vi "final.reaction method and 1ST ziegler method).vi"() -> ()   [LabVIEW 2021]
uses:
  <vilib>/addons/Control Design/_Model Construction/Model Typedefs.llb/CD Transfer Function Model (MIMO).ctl
  <vilib>/addons/Control Design/_Model Construction/Model Typedefs.llb/CD General Elements.ctl
  <vilib>/addons/Control Design/_Model Construction/Model Typedefs.llb/CD Transfer Function Model (SISO).ctl
  <vilib>/addons/Control Design/_Model Construction/Special Model Creation.llb/Special Model Creation SubVI/CD Create PID Academic Model.vi
  <vilib>/addons/Control Design/_Dynamic Analysis/Dynamic Analysis.llb/Dynamic Analysis subVI/cd_Root Locus (Transfer Function).vi
  <vilib>/addons/Control Design/_Model Interconnection/Model Interconnection.llb/Model Interconnection SubVI/cd_Feedback (TF and TF).vi
  <vilib>/addons/Control Design/_Time Response Analysis/Time Response.llb/Time Response subVI/cd_Step Response (Transfer Function).vi
  <vilib>/addons/Control Design/_Model Construction/Model Creation.llb/Model Creation SubVI/cd_Create Transfer Function Model.vi
  <vilib>/addons/Control Design/_Model Interconnection/Model Interconnection.llb/Model Interconnection SubVI/cd_Matrix Multiply Models (TF and TF).vi
  <vilib>/addons/Control Design/_Utility/Model Viewer.llb/Model Viewer SubVI/cd_Draw Transfer Function Equation (TF).vi
  <vilib>/addons/Control Design/_Model Construction/NI_CD_Special Model Creation.lvlib
  <vilib>/addons/Control Design/_Model Interconnection/NI_CD_Model Interconnection.lvlib
  <vilib>/addons/Control Design/_Dynamic Analysis/NI_CD_Dynamic Analysis.lvlib
  <vilib>/addons/Control Design/_Time Response Analysis/NI_CD_Time Response.lvlib
  <vilib>/addons/Control Design/_Model Construction/NI_LinSys_Model Creation.lvlib
  <vilib>/addons/Control Design/_Utility/NI_CD_Model Viewer.lvlib
  <vilib>/addons/Control Design/_Model Construction/NI_LinSys_Model Typedefs.lvlib
panel:
  in  "Ti":dbl
  in  "Td":dbl
  in  "Kp":dbl
  in  "Td":dbl
  in  "Ti":dbl
  in  "Kp":dbl
  out "Root Locus G 2":cluster{dbl[], dbl[]}[](graph)=[{[], []}, {[-0.32653061224489793], [0.0]}, {[], []}, {[], []}, {array[437 elements], [0.0, 0.0, 0.0, 0.0, 0.0, 0.0, 0.0, 0.0, 0.0, 0.0, 0.0, 0.0, 0.0, 0.0, 0.0, 0.0, 0.0, 0.0, 0.0, 0.0, 0.0, 0.0, 0.0, 0.0, 0.0, 0.0, 0.0, 0.0, 0.0, 0.0, 0.0, 0.0, 0.0, 0.0, 0.0, 0.0, 0.0, 0.0, 0.0, 0.0, 0.0, 0.0, 0.0, 0.0, 0.0, 0.0, 0.0, 0.0, 0.0, 0.0, 0.0, 0.0, 0.0, 0.0, 0.0, 0.0, 0.0, 0.0, 0.0, 0.0, 0.0, 0.0, 0.0, 0.0, 0.0, 0.0, 0.0, 0.0, 0.0, 0.0, 0.0, 0.0, 0.0, 0.0, 0.0, 0.0, 0.0, 0.0, 0.0, 0.0, 0.0, 0.0, 0.0, 0.0, 0.0, 0.0, 0.0, 0.0, 0.0, 0.0, 0.0, 0.0, 0.0, 0.0, 0.0, 0.0, 0.0, 0.0, 0.0, 0.0, 0.0, 0.0, 0.0, 0.0, 0.0, 0.0, 0.0, 0.0, 0.0, 0.0, 0.0, 0.0, 0.0, 0.0, 0.0, 0.0, 0.0, 0.0, 0.0, 0.0, 0.0, 0.0, 0.0, 0.0, 0.0, 0.0, 0.0, 0.0, 0.0, 0.0, 0.0, 0.0, 0.0, 0.0, 0.0, 0.0, 0.0, 0.0, 0.0, 0.0, 0.0, 0.0, 0.0, 0.0, 0.0, 0.0, 0.0, 0.0, 0.0, 0.0, 0.0, 0.0, 0.0, 0.0, 0.0, 0.0, 0.0, 0.0, 0.0, 0.0, 0.0, 0.0, 0.0, 0.0, 0.0, 0.0, 0.0, 0.0, 0.0, 0.0, 0.0, 0.0, 0.0, 0.0, 0.0, 0.0, 0.0, 0.0, 0.0, 0.0, 0.0, 0.0, 0.0, 0.0, 0.0, 0.0, 0.0, 0.0, 0.0, 0.0, 0.0, 0.0, 0.0, 0.0, 0.0, 0.0, 0.0, 0.0, 0.0, 0.0, 0.0, 0.0, 0.0, 0.0, 0.0, 0.0, 0.0, 0.0, 0.0, 0.0, 0.0, 0.0, 0.0, 0.0, 0.0, 0.0, 0.0, 0.0, 0.0, 0.0, 0.0, 0.0, 0.0, 0.0, 0.0, 0.0, 0.0, 0.0, 0.0, 0.0, 0.0, 0.0, 0.0, 0.0, 0.0, 0.0, 0.0, 0.0, 0.0, 0.0, 0.0, 0.0, 0.0, 0.0, 0.0, 0.0, 0.0, 0.0, 0.0, 0.0, 0.0, 0.0, 0.0, 0.0, 0.0, 0.0, 0.0, 0.0, 0.0, 0.0, 0.0, 0.0, 0.0, 0.0, 0.0, 0.0, 0.0, 0.0, 0.0, 0.0, 0.0, 0.0, 0.0, 0.0, 0.0, 0.0, 0.0, 0.0, 0.0, 0.0, 0.0, 0.0, 0.0, 0.0, 0.0, 0.0, nan, nan, nan, nan, nan, nan, nan, nan, nan, nan, nan, nan, nan, nan, nan, nan, nan, nan, nan, nan, nan, nan, nan, nan, nan, nan, nan, nan, nan, nan, nan, nan, nan, nan, nan, nan, nan, nan, nan, nan, nan, nan, nan, nan, nan, nan, nan, nan, nan, nan, nan, nan, nan, nan, nan, nan, nan, nan, nan, nan, nan, nan, nan, nan, nan, nan, nan, nan, nan, nan, nan, nan, nan, nan, nan, nan, nan, nan, nan, nan, nan, nan, nan, nan, nan, nan, nan, nan, nan, nan, nan, nan, nan, nan, nan, nan, nan, nan, nan, nan, nan, nan, nan, nan, nan, nan, nan, nan, nan, nan, nan, nan, nan, nan, nan, nan, nan, nan, nan, nan, nan, nan, nan, nan, nan, nan, nan, nan, nan, nan, nan, nan, nan, nan, nan, nan, nan, nan, nan, nan, nan, nan, nan, nan, nan, nan, nan, nan, nan, nan, nan]}]
  out "Ramp Response PID  2":cluster{"time":dbl[], dbl[]}[](graph)=[{"time"=[0.0, 0.3093434343434344, 0.6186868686868688, 0.9280303030303032, 1.2373737373737377, 1.5467171717171722, 1.8560606060606064, 2.165404040404041, 2.4747474747474754, 2.7840909090909096, 3.0934343434343443, 3.4027777777777786, 3.712121212121213, 4.021464646464647, 4.330808080808082, 4.6401515151515165, 4.949494949494951, 5.258838383838385, 5.568181818181819, 5.877525252525254, 6.186868686868689, 6.496212121212123, 6.805555555555557, 7.114898989898991, 7.424242424242426, 7.733585858585861, 8.042929292929294, 8.35227272727273, 8.661616161616164, 8.970959595959599, 9.280303030303033, 9.589646464646467, 9.898989898989901, 10.208333333333336, 10.51767676767677, 10.827020202020204, 11.136363636363638, 11.445707070707073, 11.755050505050509, 12.064393939393943, 12.373737373737377], [0.0, 0.08971912221391998, 0.16317492670961967, 0.22331545284233406, 0.27255435109347836, 0.31286775133936867, 0.3458735718818212, 0.37289645219050066, 0.39502091533596234, 0.4131348937084926, 0.42796536486267295, 0.44010752767923655, 0.4500486897860373, 0.45818782492420873, 0.46485158516528746, 0.47030741060579706, 0.47477426267736766, 0.4784314118378126, 0.48142563232406227, 0.48387709271765095, 0.4858841787318348, 0.4875274417757199, 0.48887283176514507, 0.4899743439243708, 0.4908761858040183, 0.4916145514852993, 0.4922190741755815, 0.4927140154930489, 0.4931192391706285, 0.4934510082573383, 0.4937226378115482, 0.49394502928102463, 0.49412710801630716, 0.4942761814763646, 0.49439823250258136, 0.4944981594311897, 0.4945799726807021, 0.494646955704087, 0.4947017967652665, 0.4947466968285855, 0.49478345789124]}, {"time"=[0.0, 0.11874999999999998, 0.23749999999999996, 0.35624999999999996, 0.4749999999999999, 0.5937499999999999, 0.7124999999999999, 0.8312499999999998, 0.9499999999999998, 1.0687499999999999, 1.1874999999999998, 1.3062499999999997, 1.4249999999999998, 1.5437499999999997, 1.6624999999999996, 1.7812499999999998, 1.8999999999999997, 2.01875, 2.1374999999999997, 2.2562499999999996, 2.3749999999999996, 2.4937499999999995, 2.6124999999999994, 2.7312499999999997, 2.8499999999999996, 2.9687499999999996, 3.0874999999999995, 3.2062499999999994, 3.3249999999999993, 3.4437499999999996, 3.5624999999999996, 3.6812499999999995, 3.7999999999999994, 3.9187499999999993, 4.0375, 4.156249999999999, 4.2749999999999995], [0.0, 0.0, 0.0, 0.0, 0.0, 0.0, 0.0, 0.0, 0.0, 0.0, 0.0, 0.04674701942045699, 0.09781428470953771, 0.1530352107469137, 0.21224412599490042, 0.2752767774451205, 0.34197078280045506, 0.4121660332631972, 0.485705050158154, 0.562433298479174, 0.6421994603095471, 0.724855670931194, 0.8102577203047987, 0.8982652224732375, 0.9887417553140145, 1.0815549729430756, 1.1765766929524732, 1.2736829605479854, 1.3727540915400525, 1.4736746960323288, 1.5763336845467992, 1.6806242582228204, 1.786443884629593, 1.8936942606374882, 2.0022812637032796, 2.112114892837669, 2.2231092004405006]}, {"time"=[0.0, 0.01, 0.02, 0.03, 0.04, 0.05, 0.06, 0.07, 0.08, 0.09, 0.1, 0.11, 0.12, 0.13, 0.14, 0.15, 0.16, 0.17, 0.18, 0.19, 0.2, 0.21, 0.22, 0.23, 0.24, 0.25, 0.26, 0.27, 0.28, 0.29, 0.3, 0.31, 0.32, 0.33, 0.34, 0.35000000000000003, 0.36, 0.37, 0.38, 0.39, 0.4, 0.41000000000000003, 0.42, 0.43, 0.44, 0.45, 0.46, 0.47000000000000003, 0.48, 0.49, 0.5, 0.51, 0.52, 0.53, 0.54, 0.55, 0.56, 0.5700000000000001, 0.58, 0.59, 0.6, 0.61, 0.62, 0.63, 0.64, 0.65, 0.66, 0.67, 0.68, 0.6900000000000001, 0.7000000000000001, 0.71, 0.72, 0.73, 0.74, 0.75, 0.76, 0.77, 0.78, 0.79, 0.8, 0.81, 0.8200000000000001, 0.8300000000000001, 0.84, 0.85, 0.86, 0.87, 0.88, 0.89, 0.9, 0.91, 0.92, 0.93, 0.9400000000000001, 0.9500000000000001, 0.96, 0.97, 0.98, 0.99, 1.0, 1.01, 1.02, 1.03, 1.04, 1.05, 1.06, 1.07, 1.08, 1.09, 1.1, 1.11, 1.12, 1.1300000000000001, 1.1400000000000001, 1.1500000000000001, 1.16, 1.17, 1.18, 1.19, 1.2, 1.21, 1.22, 1.23, 1.24, 1.25, 1.26, 1.27, 1.28, 1.29, 1.3, 1.31, 1.32, 1.33, 1.34, 1.35, 1.36, 1.37, 1.3800000000000001, 1.3900000000000001, 1.4000000000000001, 1.41, 1.42, 1.43, 1.44, 1.45, 1.46, 1.47, 1.48, 1.49, 1.5, 1.51, 1.52, 1.53, 1.54, 1.55, 1.56, 1.57, 1.58, 1.59, 1.6, 1.61, 1.62, 1.6300000000000001, 1.6400000000000001, 1.6500000000000001, 1.6600000000000001, 1.67, 1.68, 1.69, 1.7, 1.71, 1.72, 1.73, 1.74, 1.75, 1.76, 1.77, 1.78, 1.79, 1.8, 1.81, 1.82, 1.83, 1.84, 1.85, 1.86, 1.87, 1.8800000000000001, 1.8900000000000001, 1.9000000000000001, 1.9100000000000001, 1.92, 1.93, 1.94, 1.95, 1.96, 1.97, 1.98, 1.99, 2.0, 2.0100000000000002, 2.02, 2.0300000000000002, 2.04, 2.05, 2.06, 2.07, 2.08, 2.09, 2.1, 2.11, 2.12, 2.13, 2.14, 2.15, 2.16, 2.17, 2.18, 2.19, 2.2, 2.21, 2.22, 2.23, 2.24, 2.25, 2.2600000000000002, 2.27, 2.2800000000000002, 2.29, 2.3000000000000003, 2.31, 2.32, 2.33, 2.34, 2.35, 2.36, 2.37, 2.38, 2.39, 2.4, 2.41, 2.42, 2.43, 2.44, 2.45, 2.46, 2.47, 2.48, 2.49, 2.5, 2.5100000000000002, 2.52, 2.5300000000000002, 2.54, 2.5500000000000003, 2.56, 2.57, 2.58, 2.59, 2.6, 2.61, 2.62, 2.63, 2.64, 2.65, 2.66, 2.67, 2.68, 2.69, 2.7, 2.71, 2.72, 2.73, 2.74, 2.75, 2.7600000000000002, 2.77, 2.7800000000000002, 2.79, 2.8000000000000003, 2.81, 2.82, 2.83, 2.84, 2.85, 2.86, 2.87, 2.88, 2.89, 2.9, 2.91, 2.92, 2.93, 2.94, 2.95, 2.96, 2.97, 2.98, 2.99, 3.0], [0.0, 0.01, 0.02, 0.03, 0.04, 0.05, 0.060000000000000005, 0.07, 0.08, 0.09, 0.09999999999999999, 0.10999999999999999, 0.11999999999999998, 0.12999999999999998, 0.13999999999999999, 0.15, 0.16, 0.17, 0.18000000000000002, 0.19000000000000003, 0.20000000000000004, 0.21000000000000005, 0.22000000000000006, 0.23000000000000007, 0.24000000000000007, 0.25000000000000006, 0.26000000000000006, 0.2700000000000001, 0.2800000000000001, 0.2900000000000001, 0.3000000000000001, 0.3100000000000001, 0.3200000000000001, 0.3300000000000001, 0.34000000000000014, 0.35000000000000014, 0.36000000000000015, 0.37000000000000016, 0.38000000000000017, 0.3900000000000002, 0.4000000000000002, 0.4100000000000002, 0.4200000000000002, 0.4300000000000002, 0.4400000000000002, 0.45000000000000023, 0.46000000000000024, 0.47000000000000025, 0.48000000000000026, 0.49000000000000027, 0.5000000000000002, 0.5100000000000002, 0.5200000000000002, 0.5300000000000002, 0.5400000000000003, 0.5500000000000003, 0.5600000000000003, 0.5700000000000003, 0.5800000000000003, 0.5900000000000003, 0.6000000000000003, 0.6100000000000003, 0.6200000000000003, 0.6300000000000003, 0.6400000000000003, 0.6500000000000004, 0.6600000000000004, 0.6700000000000004, 0.6800000000000004, 0.6900000000000004, 0.7000000000000004, 0.7100000000000004, 0.7200000000000004, 0.7300000000000004, 0.7400000000000004, 0.7500000000000004, 0.7600000000000005, 0.7700000000000005, 0.7800000000000005, 0.7900000000000005, 0.8000000000000005, 0.8100000000000005, 0.8200000000000005, 0.8300000000000005, 0.8400000000000005, 0.8500000000000005, 0.8600000000000005, 0.8700000000000006, 0.8800000000000006, 0.8900000000000006, 0.9000000000000006, 0.9100000000000006, 0.9200000000000006, 0.9300000000000006, 0.9400000000000006, 0.9500000000000006, 0.9600000000000006, 0.9700000000000006, 0.9800000000000006, 0.9900000000000007, 1.0000000000000007, 1.0100000000000007, 1.0200000000000007, 1.0300000000000007, 1.0400000000000007, 1.0500000000000007, 1.0600000000000007, 1.0700000000000007, 1.0800000000000007, 1.0900000000000007, 1.1000000000000008, 1.1100000000000008, 1.1200000000000008, 1.1300000000000008, 1.1400000000000008, 1.1500000000000008, 1.1600000000000008, 1.1700000000000008, 1.1800000000000008, 1.1900000000000008, 1.2000000000000008, 1.2100000000000009, 1.2200000000000009, 1.2300000000000009, 1.2400000000000009, 1.2500000000000009, 1.260000000000001, 1.270000000000001, 1.280000000000001, 1.290000000000001, 1.300000000000001, 1.310000000000001, 1.320000000000001, 1.330000000000001, 1.340000000000001, 1.350000000000001, 1.360000000000001, 1.370000000000001, 1.380000000000001, 1.390000000000001, 1.400000000000001, 1.410000000000001, 1.420000000000001, 1.430000000000001, 1.440000000000001, 1.450000000000001, 1.460000000000001, 1.470000000000001, 1.480000000000001, 1.490000000000001, 1.500000000000001, 1.5100000000000011, 1.5200000000000011, 1.5300000000000011, 1.5400000000000011, 1.5500000000000012, 1.5600000000000012, 1.5700000000000012, 1.5800000000000012, 1.5900000000000012, 1.6000000000000012, 1.6100000000000012, 1.6200000000000012, 1.6300000000000012, 1.6400000000000012, 1.6500000000000012, 1.6600000000000013, 1.6700000000000013, 1.6800000000000013, 1.6900000000000013, 1.7000000000000013, 1.7100000000000013, 1.7200000000000013, 1.7300000000000013, 1.7400000000000013, 1.7500000000000013, 1.7600000000000013, 1.7700000000000014, 1.7800000000000014, 1.7900000000000014, 1.8000000000000014, 1.8100000000000014, 1.8200000000000014, 1.8300000000000014, 1.8400000000000014, 1.8500000000000014, 1.8600000000000014, 1.8700000000000014, 1.8800000000000014, 1.8900000000000015, 1.9000000000000015, 1.9100000000000015, 1.9200000000000015, 1.9300000000000015, 1.9400000000000015, 1.9500000000000015, 1.9600000000000015, 1.9700000000000015, 1.9800000000000015, 1.9900000000000015, 2.0000000000000013, 2.010000000000001, 2.020000000000001, 2.0300000000000007, 2.0400000000000005, 2.0500000000000003, 2.06, 2.07, 2.0799999999999996, 2.0899999999999994, 2.099999999999999, 2.109999999999999, 2.1199999999999988, 2.1299999999999986, 2.1399999999999983, 2.149999999999998, 2.159999999999998, 2.1699999999999977, 2.1799999999999975, 2.1899999999999973, 2.199999999999997, 2.209999999999997, 2.2199999999999966, 2.2299999999999964, 2.239999999999996, 2.249999999999996, 2.259999999999996, 2.2699999999999956, 2.2799999999999954, 2.289999999999995, 2.299999999999995, 2.3099999999999947, 2.3199999999999945, 2.3299999999999943, 2.339999999999994, 2.349999999999994, 2.3599999999999937, 2.3699999999999934, 2.3799999999999932, 2.389999999999993, 2.399999999999993, 2.4099999999999926, 2.4199999999999924, 2.429999999999992, 2.439999999999992, 2.4499999999999917, 2.4599999999999915, 2.4699999999999913, 2.479999999999991, 2.489999999999991, 2.4999999999999907, 2.5099999999999905, 2.5199999999999902, 2.52999999999999, 2.53999999999999, 2.5499999999999896, 2.5599999999999894, 2.569999999999989, 2.579999999999989, 2.5899999999999888, 2.5999999999999885, 2.6099999999999883, 2.619999999999988, 2.629999999999988, 2.6399999999999877, 2.6499999999999875, 2.6599999999999873, 2.669999999999987, 2.679999999999987, 2.6899999999999866, 2.6999999999999864, 2.709999999999986, 2.719999999999986, 2.7299999999999858, 2.7399999999999856, 2.7499999999999853, 2.759999999999985, 2.769999999999985, 2.7799999999999847, 2.7899999999999845, 2.7999999999999843, 2.809999999999984, 2.819999999999984, 2.8299999999999836, 2.8399999999999834, 2.849999999999983, 2.859999999999983, 2.869999999999983, 2.8799999999999826, 2.8899999999999824, 2.899999999999982, 2.909999999999982, 2.9199999999999817, 2.9299999999999815, 2.9399999999999813, 2.949999999999981, 2.959999999999981, 2.9699999999999807, 2.9799999999999804, 2.9899999999999802, 2.99999999999998]}]
  out "Step Response PID 2":cluster{"time":dbl[], dbl[]}[](graph)=[{"time"=[0.0, 0.3093434343434344, 0.6186868686868688, 0.9280303030303032, 1.2373737373737377, 1.5467171717171722, 1.8560606060606064, 2.165404040404041, 2.4747474747474754, 2.7840909090909096, 3.0934343434343443, 3.4027777777777786, 3.712121212121213, 4.021464646464647, 4.330808080808082, 4.6401515151515165, 4.949494949494951, 5.258838383838385, 5.568181818181819, 5.877525252525254, 6.186868686868689, 6.496212121212123, 6.805555555555557, 7.114898989898991, 7.424242424242426, 7.733585858585861, 8.042929292929294, 8.35227272727273, 8.661616161616164, 8.970959595959599, 9.280303030303033, 9.589646464646467, 9.898989898989901, 10.208333333333336, 10.51767676767677, 10.827020202020204, 11.136363636363638, 11.445707070707073, 11.755050505050509, 12.064393939393943, 12.373737373737377], [0.0, 0.08971912221391998, 0.16317492670961967, 0.22331545284233406, 0.27255435109347836, 0.31286775133936867, 0.3458735718818212, 0.37289645219050066, 0.39502091533596234, 0.4131348937084926, 0.42796536486267295, 0.44010752767923655, 0.4500486897860373, 0.45818782492420873, 0.46485158516528746, 0.47030741060579706, 0.47477426267736766, 0.4784314118378126, 0.48142563232406227, 0.48387709271765095, 0.4858841787318348, 0.4875274417757199, 0.48887283176514507, 0.4899743439243708, 0.4908761858040183, 0.4916145514852993, 0.4922190741755815, 0.4927140154930489, 0.4931192391706285, 0.4934510082573383, 0.4937226378115482, 0.49394502928102463, 0.49412710801630716, 0.4942761814763646, 0.49439823250258136, 0.4944981594311897, 0.4945799726807021, 0.494646955704087, 0.4947017967652665, 0.4947466968285855, 0.49478345789124]}, {"time"=[0.0, 0.11874999999999998, 0.23749999999999996, 0.35624999999999996, 0.4749999999999999, 0.5937499999999999, 0.7124999999999999, 0.8312499999999998, 0.9499999999999998, 1.0687499999999999, 1.1874999999999998, 1.3062499999999997, 1.4249999999999998, 1.5437499999999997, 1.6624999999999996, 1.7812499999999998, 1.8999999999999997, 2.01875, 2.1374999999999997, 2.2562499999999996, 2.3749999999999996, 2.4937499999999995, 2.6124999999999994, 2.7312499999999997, 2.8499999999999996, 2.9687499999999996, 3.0874999999999995, 3.2062499999999994, 3.3249999999999993, 3.4437499999999996, 3.5624999999999996, 3.6812499999999995, 3.7999999999999994, 3.9187499999999993, 4.0375, 4.156249999999999, 4.2749999999999995, 4.393749999999999, 4.512499999999999, 4.63125, 4.749999999999999, 4.8687499999999995, 4.987499999999999, 5.106249999999999, 5.224999999999999, 5.343749999999999, 5.4624999999999995, 5.581249999999999, 5.699999999999999, 5.818749999999999, 5.937499999999999, 6.056249999999999, 6.174999999999999, 6.293749999999999, 6.412499999999999, 6.531249999999999, 6.649999999999999, 6.768749999999999, 6.887499999999999, 7.006249999999999, 7.124999999999999, 7.243749999999999, 7.362499999999999, 7.481249999999998, 7.599999999999999, 7.718749999999999, 7.837499999999999, 7.956249999999999, 8.075, 8.193749999999998, 8.312499999999998, 8.431249999999999, 8.549999999999999, 8.66875, 8.787499999999998, 8.906249999999998, 9.024999999999999, 9.143749999999999, 9.2625, 9.381249999999998, 9.499999999999998, 9.618749999999999, 9.737499999999999, 9.856249999999998, 9.974999999999998, 10.093749999999998, 10.212499999999999, 10.331249999999999, 10.449999999999998, 10.568749999999998, 10.687499999999998, 10.806249999999999, 10.924999999999999, 11.043749999999998, 11.162499999999998, 11.281249999999998, 11.399999999999999, 11.518749999999999, 11.637499999999998, 11.756249999999998, 11.874999999999998, 11.993749999999999, 12.112499999999997, 12.231249999999998, 12.349999999999998, 12.468749999999998, 12.587499999999999, 12.706249999999997, 12.824999999999998, 12.943749999999998, 13.062499999999998, 13.181249999999999, 13.299999999999997, 13.418749999999998, 13.537499999999998, 13.656249999999998, 13.774999999999999, 13.893749999999997, 14.012499999999998, 14.131249999999998, 14.249999999999998, 14.368749999999997, 14.487499999999997, 14.606249999999998, 14.724999999999998, 14.843749999999998, 14.962499999999997, 15.081249999999997, 15.199999999999998, 15.318749999999998, 15.437499999999998, 15.556249999999997, 15.674999999999997, 15.793749999999998, 15.912499999999998, 16.031249999999996, 16.15, 16.268749999999997, 16.387499999999996, 16.506249999999998, 16.624999999999996, 16.74375, 16.862499999999997, 16.981249999999996, 17.099999999999998, 17.218749999999996, 17.3375, 17.456249999999997, 17.574999999999996, 17.693749999999998, 17.812499999999996, 17.93125, 18.049999999999997, 18.168749999999996, 18.287499999999998, 18.406249999999996, 18.525, 18.643749999999997, 18.762499999999996, 18.881249999999998, 18.999999999999996, 19.11875, 19.237499999999997, 19.356249999999996, 19.474999999999998, 19.593749999999996, 19.712499999999995, 19.831249999999997, 19.949999999999996, 20.068749999999998, 20.187499999999996, 20.306249999999995, 20.424999999999997], [0.0, 0.0, 0.0, 0.0, 0.0, 0.0, 0.0, 0.0, 0.0, 0.0, 0.37499999999999994, 0.41208383650020264, 0.4477625386272583, 0.4820415181676434, 0.5149306710217187, 0.546443918273478, 0.5765987762501894, 0.60541595436764, 0.6329189795713029, 0.659133846201218, 0.6840886901283811, 0.7078134860326692, 0.7303397667164837, 0.7517003633741237, 0.7719291657641358, 0.7910609012603143, 0.8091309317864142, 0.826175067669815, 0.8422293974801205, 0.8573301329498857, 0.871513468106107, 0.8848154517727276, 0.8972718726360158, 0.9089181560961823, 0.9197892721599139, 0.9299196536595047, 0.9393431241148937, 0.9480928345850927, 0.9562012088851455, 0.9636998965738381, 0.9706197331458364, 0.9769907068897197, 0.9828419319004598, 0.9882016267612508, 0.9930970984351859, 0.9975547309321007, 1.0015999783399123, 1.005257361833018, 1.008550470292714, 1.0115019641961918, 1.014133582451457, 1.0164661518754707, 1.018519599031985, 1.0203129641639086, 1.0218644169726037, 1.0231912740133304, 1.0243100174920705, 1.0252363152642676, 1.025985041850562, 1.0265703002984465, 1.027005444731907, 1.027303103443579, 1.0274752023957554, 1.0275329890077547, 1.0274870561176976, 1.0273473660167067, 1.027123274462909, 1.0268235545914517, 1.0264564206450182, 1.0260295514571196, 1.0255501136277019, 1.0250247843374294, 1.0244597737533598, 1.0238608469846466, 1.0232333455524238, 1.0225822083431462, 1.0219119920194026, 1.021226890866614, 1.020530756058076, 1.0198271143245452, 1.0191191860179887, 1.0184099025622688, 1.0177019232863962, 1.016997651638608, 1.0162992507818982, 1.0156086585737762, 1.014927601934967, 1.014257610613496, 1.0136000303521622, 1.0129560354687606, 1.0123266408596414, 1.0117127134382407, 1.0111149830211406, 1.0105340526749993, 1.0099704085383578, 1.0094244291328764, 1.0088963941790066, 1.008386492931452, 1.0078948320500378, 1.007421443021783, 1.006966289150093, 1.0065292721270185, 1.006110238204514, 1.0057089839805538, 1.0053252618158426, 1.004958784896684, 1.0046092319593687, 1.0042762516911932, 1.0039594668229592, 1.0036584779274862, 1.0033728669383584, 1.0031022004027752, 1.002846032482018, 1.0026039077126674, 1.0023753635413133, 1.00215993264512, 1.0019571450501852, 1.00176653005924, 1.0015876179998215, 1.0014199418036387, 1.0012630384274408, 1.0011164501252932, 1.0009797255817554, 1.000852420915059, 1.0007341005589863, 1.0006243380317605, 1.00052271659988, 1.0004288298444477, 1.0003422821371901, 1.0002626890329978, 1.0001896775854693, 1.0001228865916116, 1.0000619667715123, 1.0000065808884857, 0.9999564038148911, 0.9999111225485162, 0.9998704361841395, 0.9998340558446084, 0.9998017045755001, 0.9997731172071864, 0.9997480401878693, 0.9997262313909276, 0.9997074598996916, 0.9996915057725395, 0.9996781597910218, 0.9996672231935075, 0.9996585073966762, 0.9996518337069942, 0.999647033024156, 0.9996439455383013, 0.9996424204226821, 0.9996423155233032, 0.9996434970469326, 0.9996458392487444, 0.9996492241207497, 0.9996535410820484, 0.9996586866718364, 0.9996645642460062, 0.9996710836780791, 0.9996781610651322, 0.9996857184392944, 0.9996936834853181, 0.9997019892646546, 0.9997105739464132, 0.9997193805455022, 0.9997283566682198, 0.9997374542654873, 0.9997466293938946, 0.9997558419846626, 0.999765055620607, 0.9997742373211389, 0.9997833573353125, 0.9997923889428968]}, {"time"=[0.0, 0.01, 0.02, 0.03, 0.04, 0.05, 0.06, 0.07, 0.08, 0.09, 0.1, 0.11, 0.12, 0.13, 0.14, 0.15, 0.16, 0.17, 0.18, 0.19, 0.2, 0.21, 0.22, 0.23, 0.24, 0.25, 0.26, 0.27, 0.28, 0.29, 0.3, 0.31, 0.32, 0.33, 0.34, 0.35000000000000003, 0.36, 0.37, 0.38, 0.39, 0.4, 0.41000000000000003, 0.42, 0.43, 0.44, 0.45, 0.46, 0.47000000000000003, 0.48, 0.49, 0.5, 0.51, 0.52, 0.53, 0.54, 0.55, 0.56, 0.5700000000000001, 0.58, 0.59, 0.6, 0.61, 0.62, 0.63, 0.64, 0.65, 0.66, 0.67, 0.68, 0.6900000000000001, 0.7000000000000001, 0.71, 0.72, 0.73, 0.74, 0.75, 0.76, 0.77, 0.78, 0.79, 0.8, 0.81, 0.8200000000000001, 0.8300000000000001, 0.84, 0.85, 0.86, 0.87, 0.88, 0.89, 0.9, 0.91, 0.92, 0.93, 0.9400000000000001, 0.9500000000000001, 0.96, 0.97, 0.98, 0.99, 1.0, 1.01, 1.02, 1.03, 1.04, 1.05, 1.06, 1.07, 1.08, 1.09, 1.1, 1.11, 1.12, 1.1300000000000001, 1.1400000000000001, 1.1500000000000001, 1.16, 1.17, 1.18, 1.19, 1.2, 1.21, 1.22, 1.23, 1.24, 1.25, 1.26, 1.27, 1.28, 1.29, 1.3, 1.31, 1.32, 1.33, 1.34, 1.35, 1.36, 1.37, 1.3800000000000001, 1.3900000000000001, 1.4000000000000001, 1.41, 1.42, 1.43, 1.44, 1.45, 1.46, 1.47, 1.48, 1.49, 1.5, 1.51, 1.52, 1.53, 1.54, 1.55, 1.56, 1.57, 1.58, 1.59, 1.6, 1.61, 1.62, 1.6300000000000001, 1.6400000000000001, 1.6500000000000001, 1.6600000000000001, 1.67, 1.68, 1.69, 1.7, 1.71, 1.72, 1.73, 1.74, 1.75, 1.76, 1.77, 1.78, 1.79, 1.8, 1.81, 1.82, 1.83, 1.84, 1.85, 1.86, 1.87, 1.8800000000000001, 1.8900000000000001, 1.9000000000000001, 1.9100000000000001, 1.92, 1.93, 1.94, 1.95, 1.96, 1.97, 1.98, 1.99, 2.0, 2.0100000000000002, 2.02, 2.0300000000000002, 2.04, 2.05, 2.06, 2.07, 2.08, 2.09, 2.1, 2.11, 2.12, 2.13, 2.14, 2.15, 2.16, 2.17, 2.18, 2.19, 2.2, 2.21, 2.22, 2.23, 2.24, 2.25, 2.2600000000000002, 2.27, 2.2800000000000002, 2.29, 2.3000000000000003, 2.31, 2.32, 2.33, 2.34, 2.35, 2.36, 2.37, 2.38, 2.39, 2.4, 2.41, 2.42, 2.43, 2.44, 2.45, 2.46, 2.47, 2.48, 2.49, 2.5, 2.5100000000000002, 2.52, 2.5300000000000002, 2.54, 2.5500000000000003, 2.56, 2.57, 2.58, 2.59, 2.6, 2.61, 2.62, 2.63, 2.64, 2.65, 2.66, 2.67, 2.68, 2.69, 2.7, 2.71, 2.72, 2.73, 2.74, 2.75, 2.7600000000000002, 2.77, 2.7800000000000002, 2.79, 2.8000000000000003, 2.81, 2.82, 2.83, 2.84, 2.85, 2.86, 2.87, 2.88, 2.89, 2.9, 2.91, 2.92, 2.93, 2.94, 2.95, 2.96, 2.97, 2.98, 2.99, 3.0], [1.0, 1.0, 1.0, 1.0, 1.0, 1.0, 1.0, 1.0, 1.0, 1.0, 1.0, 1.0, 1.0, 1.0, 1.0, 1.0, 1.0, 1.0, 1.0, 1.0, 1.0, 1.0, 1.0, 1.0, 1.0, 1.0, 1.0, 1.0, 1.0, 1.0, 1.0, 1.0, 1.0, 1.0, 1.0, 1.0, 1.0, 1.0, 1.0, 1.0, 1.0, 1.0, 1.0, 1.0, 1.0, 1.0, 1.0, 1.0, 1.0, 1.0, 1.0, 1.0, 1.0, 1.0, 1.0, 1.0, 1.0, 1.0, 1.0, 1.0, 1.0, 1.0, 1.0, 1.0, 1.0, 1.0, 1.0, 1.0, 1.0, 1.0, 1.0, 1.0, 1.0, 1.0, 1.0, 1.0, 1.0, 1.0, 1.0, 1.0, 1.0, 1.0, 1.0, 1.0, 1.0, 1.0, 1.0, 1.0, 1.0, 1.0, 1.0, 1.0, 1.0, 1.0, 1.0, 1.0, 1.0, 1.0, 1.0, 1.0, 1.0, 1.0, 1.0, 1.0, 1.0, 1.0, 1.0, 1.0, 1.0, 1.0, 1.0, 1.0, 1.0, 1.0, 1.0, 1.0, 1.0, 1.0, 1.0, 1.0, 1.0, 1.0, 1.0, 1.0, 1.0, 1.0, 1.0, 1.0, 1.0, 1.0, 1.0, 1.0, 1.0, 1.0, 1.0, 1.0, 1.0, 1.0, 1.0, 1.0, 1.0, 1.0, 1.0, 1.0, 1.0, 1.0, 1.0, 1.0, 1.0, 1.0, 1.0, 1.0, 1.0, 1.0, 1.0, 1.0, 1.0, 1.0, 1.0, 1.0, 1.0, 1.0, 1.0, 1.0, 1.0, 1.0, 1.0, 1.0, 1.0, 1.0, 1.0, 1.0, 1.0, 1.0, 1.0, 1.0, 1.0, 1.0, 1.0, 1.0, 1.0, 1.0, 1.0, 1.0, 1.0, 1.0, 1.0, 1.0, 1.0, 1.0, 1.0, 1.0, 1.0, 1.0, 1.0, 1.0, 1.0, 1.0, 1.0, 1.0, 1.0, 1.0, 1.0, 1.0, 1.0, 1.0, 1.0, 1.0, 1.0, 1.0, 1.0, 1.0, 1.0, 1.0, 1.0, 1.0, 1.0, 1.0, 1.0, 1.0, 1.0, 1.0, 1.0, 1.0, 1.0, 1.0, 1.0, 1.0, 1.0, 1.0, 1.0, 1.0, 1.0, 1.0, 1.0, 1.0, 1.0, 1.0, 1.0, 1.0, 1.0, 1.0, 1.0, 1.0, 1.0, 1.0, 1.0, 1.0, 1.0, 1.0, 1.0, 1.0, 1.0, 1.0, 1.0, 1.0, 1.0, 1.0, 1.0, 1.0, 1.0, 1.0, 1.0, 1.0, 1.0, 1.0, 1.0, 1.0, 1.0, 1.0, 1.0, 1.0, 1.0, 1.0, 1.0, 1.0, 1.0, 1.0, 1.0, 1.0, 1.0, 1.0, 1.0, 1.0, 1.0, 1.0, 1.0, 1.0, 1.0, 1.0, 1.0, 1.0, 1.0, 1.0, 1.0, 1.0, 1.0, 1.0, 1.0, 1.0, 1.0]}]
  out "Root Locus PID 2":cluster{dbl[], dbl[]}[](graph)=[{[], []}, {[-0.32653061224489793, 0.0], [0.0, 0.0]}, {[-0.8421052631578949, -0.8421052631578949], [1.1468530207045996e-08, -1.1468530207045996e-08]}, {[-0.20253164556962014], [0.0]}, {array[413 elements], array[413 elements]}, {array[413 elements], array[413 elements]}]
  out "Equation":picture
  out "open loop step response":cluster{"time":dbl[], dbl[]}[](graph)=[{"time"=array[218 elements], array[218 elements]}, {"time"=[0.0, 0.01, 0.02, 0.03, 0.04, 0.05, 0.06, 0.07, 0.08, 0.09, 0.1, 0.11, 0.12, 0.13, 0.14, 0.15, 0.16, 0.17, 0.18, 0.19, 0.2, 0.21, 0.22, 0.23, 0.24, 0.25, 0.26, 0.27, 0.28, 0.29, 0.3, 0.31, 0.32, 0.33, 0.34, 0.35000000000000003, 0.36, 0.37, 0.38, 0.39, 0.4, 0.41000000000000003, 0.42, 0.43, 0.44, 0.45, 0.46, 0.47000000000000003, 0.48, 0.49, 0.5, 0.51, 0.52, 0.53, 0.54, 0.55, 0.56, 0.5700000000000001, 0.58, 0.59, 0.6, 0.61, 0.62, 0.63, 0.64, 0.65, 0.66, 0.67, 0.68, 0.6900000000000001, 0.7000000000000001, 0.71, 0.72, 0.73, 0.74, 0.75, 0.76, 0.77, 0.78, 0.79, 0.8, 0.81, 0.8200000000000001, 0.8300000000000001, 0.84, 0.85, 0.86, 0.87, 0.88, 0.89, 0.9, 0.91, 0.92, 0.93, 0.9400000000000001, 0.9500000000000001, 0.96, 0.97, 0.98, 0.99, 1.0, 1.01, 1.02, 1.03, 1.04, 1.05, 1.06, 1.07, 1.08, 1.09, 1.1, 1.11, 1.12, 1.1300000000000001, 1.1400000000000001, 1.1500000000000001, 1.16, 1.17, 1.18, 1.19, 1.2, 1.21, 1.22, 1.23, 1.24, 1.25, 1.26, 1.27, 1.28, 1.29, 1.3, 1.31, 1.32, 1.33, 1.34, 1.35, 1.36, 1.37, 1.3800000000000001, 1.3900000000000001, 1.4000000000000001, 1.41, 1.42, 1.43, 1.44, 1.45, 1.46, 1.47, 1.48, 1.49, 1.5, 1.51, 1.52, 1.53, 1.54, 1.55, 1.56, 1.57, 1.58, 1.59, 1.6, 1.61, 1.62, 1.6300000000000001, 1.6400000000000001, 1.6500000000000001, 1.6600000000000001, 1.67, 1.68, 1.69, 1.7, 1.71, 1.72, 1.73, 1.74, 1.75, 1.76, 1.77, 1.78, 1.79, 1.8, 1.81, 1.82, 1.83, 1.84, 1.85, 1.86, 1.87, 1.8800000000000001, 1.8900000000000001, 1.9000000000000001, 1.9100000000000001, 1.92, 1.93, 1.94, 1.95, 1.96, 1.97, 1.98, 1.99, 2.0, 2.0100000000000002, 2.02, 2.0300000000000002, 2.04, 2.05, 2.06, 2.07, 2.08, 2.09, 2.1, 2.11, 2.12, 2.13, 2.14, 2.15, 2.16, 2.17, 2.18, 2.19, 2.2, 2.21, 2.22, 2.23, 2.24, 2.25, 2.2600000000000002, 2.27, 2.2800000000000002, 2.29, 2.3000000000000003, 2.31, 2.32, 2.33, 2.34, 2.35, 2.36, 2.37, 2.38, 2.39, 2.4, 2.41, 2.42, 2.43, 2.44, 2.45, 2.46, 2.47, 2.48, 2.49, 2.5, 2.5100000000000002, 2.52, 2.5300000000000002, 2.54, 2.5500000000000003, 2.56, 2.57, 2.58, 2.59, 2.6, 2.61, 2.62, 2.63, 2.64, 2.65, 2.66, 2.67, 2.68, 2.69, 2.7, 2.71, 2.72, 2.73, 2.74, 2.75, 2.7600000000000002, 2.77, 2.7800000000000002, 2.79, 2.8000000000000003, 2.81, 2.82, 2.83, 2.84, 2.85, 2.86, 2.87, 2.88, 2.89, 2.9, 2.91, 2.92, 2.93, 2.94, 2.95, 2.96, 2.97, 2.98, 2.99, 3.0], [1.0, 1.0, 1.0, 1.0, 1.0, 1.0, 1.0, 1.0, 1.0, 1.0, 1.0, 1.0, 1.0, 1.0, 1.0, 1.0, 1.0, 1.0, 1.0, 1.0, 1.0, 1.0, 1.0, 1.0, 1.0, 1.0, 1.0, 1.0, 1.0, 1.0, 1.0, 1.0, 1.0, 1.0, 1.0, 1.0, 1.0, 1.0, 1.0, 1.0, 1.0, 1.0, 1.0, 1.0, 1.0, 1.0, 1.0, 1.0, 1.0, 1.0, 1.0, 1.0, 1.0, 1.0, 1.0, 1.0, 1.0, 1.0, 1.0, 1.0, 1.0, 1.0, 1.0, 1.0, 1.0, 1.0, 1.0, 1.0, 1.0, 1.0, 1.0, 1.0, 1.0, 1.0, 1.0, 1.0, 1.0, 1.0, 1.0, 1.0, 1.0, 1.0, 1.0, 1.0, 1.0, 1.0, 1.0, 1.0, 1.0, 1.0, 1.0, 1.0, 1.0, 1.0, 1.0, 1.0, 1.0, 1.0, 1.0, 1.0, 1.0, 1.0, 1.0, 1.0, 1.0, 1.0, 1.0, 1.0, 1.0, 1.0, 1.0, 1.0, 1.0, 1.0, 1.0, 1.0, 1.0, 1.0, 1.0, 1.0, 1.0, 1.0, 1.0, 1.0, 1.0, 1.0, 1.0, 1.0, 1.0, 1.0, 1.0, 1.0, 1.0, 1.0, 1.0, 1.0, 1.0, 1.0, 1.0, 1.0, 1.0, 1.0, 1.0, 1.0, 1.0, 1.0, 1.0, 1.0, 1.0, 1.0, 1.0, 1.0, 1.0, 1.0, 1.0, 1.0, 1.0, 1.0, 1.0, 1.0, 1.0, 1.0, 1.0, 1.0, 1.0, 1.0, 1.0, 1.0, 1.0, 1.0, 1.0, 1.0, 1.0, 1.0, 1.0, 1.0, 1.0, 1.0, 1.0, 1.0, 1.0, 1.0, 1.0, 1.0, 1.0, 1.0, 1.0, 1.0, 1.0, 1.0, 1.0, 1.0, 1.0, 1.0, 1.0, 1.0, 1.0, 1.0, 1.0, 1.0, 1.0, 1.0, 1.0, 1.0, 1.0, 1.0, 1.0, 1.0, 1.0, 1.0, 1.0, 1.0, 1.0, 1.0, 1.0, 1.0, 1.0, 1.0, 1.0, 1.0, 1.0, 1.0, 1.0, 1.0, 1.0, 1.0, 1.0, 1.0, 1.0, 1.0, 1.0, 1.0, 1.0, 1.0, 1.0, 1.0, 1.0, 1.0, 1.0, 1.0, 1.0, 1.0, 1.0, 1.0, 1.0, 1.0, 1.0, 1.0, 1.0, 1.0, 1.0, 1.0, 1.0, 1.0, 1.0, 1.0, 1.0, 1.0, 1.0, 1.0, 1.0, 1.0, 1.0, 1.0, 1.0, 1.0, 1.0, 1.0, 1.0, 1.0, 1.0, 1.0, 1.0, 1.0, 1.0, 1.0, 1.0, 1.0, 1.0, 1.0, 1.0, 1.0, 1.0, 1.0, 1.0, 1.0, 1.0, 1.0, 1.0, 1.0, 1.0, 1.0, 1.0, 1.0, 1.0, 1.0, 1.0, 1.0, 1.0, 1.0, 1.0]}]
  in  "Td":dbl
  in  "Kp":dbl
  in  "Pcr":dbl
  in  "Kcr":dbl
  in  "choose 2":string(combo)
  out "Root Locus G":cluster{dbl[], dbl[]}[](graph)
  out "Ramp Response PID":cluster{"time":dbl[], dbl[]}[](graph)=[{"time"=[0.0, 0.01, 0.02, 0.03, 0.04, 0.05, 0.06, 0.07, 0.08, 0.09, 0.1, 0.11, 0.12, 0.13, 0.14, 0.15, 0.16, 0.17, 0.18, 0.19, 0.2, 0.21, 0.22, 0.23, 0.24, 0.25, 0.26, 0.27, 0.28, 0.29, 0.3, 0.31, 0.32, 0.33, 0.34, 0.35000000000000003, 0.36, 0.37, 0.38, 0.39, 0.4, 0.41000000000000003, 0.42, 0.43, 0.44, 0.45, 0.46, 0.47000000000000003, 0.48, 0.49, 0.5, 0.51, 0.52, 0.53, 0.54, 0.55, 0.56, 0.5700000000000001, 0.58, 0.59, 0.6, 0.61, 0.62, 0.63, 0.64, 0.65, 0.66, 0.67, 0.68, 0.6900000000000001, 0.7000000000000001, 0.71, 0.72, 0.73, 0.74, 0.75, 0.76, 0.77, 0.78, 0.79, 0.8, 0.81, 0.8200000000000001, 0.8300000000000001, 0.84, 0.85, 0.86, 0.87, 0.88, 0.89, 0.9, 0.91, 0.92, 0.93, 0.9400000000000001, 0.9500000000000001, 0.96, 0.97, 0.98, 0.99, 1.0, 1.01, 1.02, 1.03, 1.04, 1.05, 1.06, 1.07, 1.08, 1.09, 1.1, 1.11, 1.12, 1.1300000000000001, 1.1400000000000001, 1.1500000000000001, 1.16, 1.17, 1.18, 1.19, 1.2, 1.21, 1.22, 1.23, 1.24, 1.25, 1.26, 1.27, 1.28, 1.29, 1.3, 1.31, 1.32, 1.33, 1.34, 1.35, 1.36, 1.37, 1.3800000000000001, 1.3900000000000001, 1.4000000000000001, 1.41, 1.42, 1.43, 1.44, 1.45, 1.46, 1.47, 1.48, 1.49, 1.5, 1.51, 1.52, 1.53, 1.54, 1.55, 1.56, 1.57, 1.58, 1.59, 1.6, 1.61, 1.62, 1.6300000000000001, 1.6400000000000001, 1.6500000000000001, 1.6600000000000001, 1.67, 1.68, 1.69, 1.7, 1.71, 1.72, 1.73, 1.74, 1.75, 1.76, 1.77, 1.78, 1.79, 1.8, 1.81, 1.82, 1.83, 1.84, 1.85, 1.86, 1.87, 1.8800000000000001, 1.8900000000000001, 1.9000000000000001, 1.9100000000000001, 1.92, 1.93, 1.94, 1.95, 1.96, 1.97, 1.98, 1.99, 2.0, 2.0100000000000002, 2.02, 2.0300000000000002, 2.04, 2.05, 2.06, 2.07, 2.08, 2.09, 2.1, 2.11, 2.12, 2.13, 2.14, 2.15, 2.16, 2.17, 2.18, 2.19, 2.2, 2.21, 2.22, 2.23, 2.24, 2.25, 2.2600000000000002, 2.27, 2.2800000000000002, 2.29, 2.3000000000000003, 2.31, 2.32, 2.33, 2.34, 2.35, 2.36, 2.37, 2.38, 2.39, 2.4, 2.41, 2.42, 2.43, 2.44, 2.45, 2.46, 2.47, 2.48, 2.49, 2.5, 2.5100000000000002, 2.52, 2.5300000000000002, 2.54, 2.5500000000000003, 2.56, 2.57, 2.58, 2.59, 2.6, 2.61, 2.62, 2.63, 2.64, 2.65, 2.66, 2.67, 2.68, 2.69, 2.7, 2.71, 2.72, 2.73, 2.74, 2.75, 2.7600000000000002, 2.77, 2.7800000000000002, 2.79, 2.8000000000000003, 2.81, 2.82, 2.83, 2.84, 2.85, 2.86, 2.87, 2.88, 2.89, 2.9, 2.91, 2.92, 2.93, 2.94, 2.95, 2.96, 2.97, 2.98, 2.99, 3.0], [0.0, 0.0, 0.0, 0.0, 0.0, 0.0, 0.0, 0.0, 0.0, 0.0, 0.0, 0.0, 0.0, 0.0, 0.0, 0.0, 0.0, 0.0, 0.0, 0.0, 0.0, 0.0, 0.0, 0.0, 0.0, 0.0, 0.0, 0.0, 0.0, 0.0, 0.0, 0.0, 0.0, 0.0, 0.0, 0.0, 0.0, 0.0, 0.0, 0.0, 0.0, 0.0, 0.0, 0.0, 0.0, 0.0, 0.0, 0.0, 0.0, 0.0, 0.0, 0.0, 0.0, 0.0, 0.0, 0.0, 0.0, 0.0, 0.0, 0.0, 0.0, 0.0, 0.0, 0.0, 0.0, 0.0, 0.0, 0.0, 0.0, 0.0, 0.0, 0.0, 0.0, 0.0, 0.0, 0.0, 0.0, 0.0, 0.0, 0.0, 0.0, 0.0, 0.0, 0.0, 0.0, 0.0, 0.0, 0.0, 0.0, 0.0, 0.0, 0.0, 0.0, 0.0, 0.0, 0.0, 0.0, 0.0, 0.0, 0.0, 0.0, 0.0, 0.0, 0.0, 0.0, 0.0, 0.0, 0.0, 0.0, 0.0, 0.0, 0.0, 0.0, 0.0, 0.0, 0.0, 0.0, 0.0, 0.0, 0.0, 0.0, 0.0, 0.0, 0.0, 0.0, 0.0, 0.0, 0.0, 0.0, 0.0, 0.0, 0.0, 0.0, 0.0, 0.0, 0.0, 0.0, 0.0, 0.0, 0.0, 0.0, 0.0, 0.0, 0.0, 0.0, 0.0, 0.0, 0.0, 0.0, 0.0, 0.0, 0.0, 0.0, 0.0, 0.0, 0.0, 0.0, 0.0, 0.0, 0.0, 0.0, 0.0, 0.0, 0.0, 0.0, 0.0, 0.0, 0.0, 0.0, 0.0, 0.0, 0.0, 0.0, 0.0, 0.0, 0.0, 0.0, 0.0, 0.0, 0.0, 0.0, 0.0, 0.0, 0.0, 0.0, 0.0, 0.0, 0.0, 0.0, 0.0, 0.0, 0.0, 0.0, 0.0, 0.0, 0.0, 0.0, 0.0, 0.0, 0.0, 0.0, 0.0, 0.0, 0.0, 0.0, 0.0, 0.0, 0.0, 0.0, 0.0, 0.0, 0.0, 0.0, 0.0, 0.0, 0.0, 0.0, 0.0, 0.0, 0.0, 0.0, 0.0, 0.0, 0.0, 0.0, 0.0, 0.0, 0.0, 0.0, 0.0, 0.0, 0.0, 0.0, 0.0, 0.0, 0.0, 0.0, 0.0, 0.0, 0.0, 0.0, 0.0, 0.0, 0.0, 0.0, 0.0, 0.0, 0.0, 0.0, 0.0, 0.0, 0.0, 0.0, 0.0, 0.0, 0.0, 0.0, 0.0, 0.0, 0.0, 0.0, 0.0, 0.0, 0.0, 0.0, 0.0, 0.0, 0.0, 0.0, 0.0, 0.0, 0.0, 0.0, 0.0, 0.0, 0.0, 0.0, 0.0, 0.0, 0.0, 0.0, 0.0, 0.0, 0.0, 0.0, 0.0, 0.0, 0.0, 0.0, 0.0, 0.0, 0.0, 0.0, 0.0, 0.0, 0.0, 0.0, 0.0, 0.0, 0.0, 0.0]}, {"time"=[0.0, 0.01, 0.02, 0.03, 0.04, 0.05, 0.06, 0.07, 0.08, 0.09, 0.1, 0.11, 0.12, 0.13, 0.14, 0.15, 0.16, 0.17, 0.18, 0.19, 0.2, 0.21, 0.22, 0.23, 0.24, 0.25, 0.26, 0.27, 0.28, 0.29, 0.3, 0.31, 0.32, 0.33, 0.34, 0.35000000000000003, 0.36, 0.37, 0.38, 0.39, 0.4, 0.41000000000000003, 0.42, 0.43, 0.44, 0.45, 0.46, 0.47000000000000003, 0.48, 0.49, 0.5, 0.51, 0.52, 0.53, 0.54, 0.55, 0.56, 0.5700000000000001, 0.58, 0.59, 0.6, 0.61, 0.62, 0.63, 0.64, 0.65, 0.66, 0.67, 0.68, 0.6900000000000001, 0.7000000000000001, 0.71, 0.72, 0.73, 0.74, 0.75, 0.76, 0.77, 0.78, 0.79, 0.8, 0.81, 0.8200000000000001, 0.8300000000000001, 0.84, 0.85, 0.86, 0.87, 0.88, 0.89, 0.9, 0.91, 0.92, 0.93, 0.9400000000000001, 0.9500000000000001, 0.96, 0.97, 0.98, 0.99, 1.0, 1.01, 1.02, 1.03, 1.04, 1.05, 1.06, 1.07, 1.08, 1.09, 1.1, 1.11, 1.12, 1.1300000000000001, 1.1400000000000001, 1.1500000000000001, 1.16, 1.17, 1.18, 1.19, 1.2, 1.21, 1.22, 1.23, 1.24, 1.25, 1.26, 1.27, 1.28, 1.29, 1.3, 1.31, 1.32, 1.33, 1.34, 1.35, 1.36, 1.37, 1.3800000000000001, 1.3900000000000001, 1.4000000000000001, 1.41, 1.42, 1.43, 1.44, 1.45, 1.46, 1.47, 1.48, 1.49, 1.5, 1.51, 1.52, 1.53, 1.54, 1.55, 1.56, 1.57, 1.58, 1.59, 1.6, 1.61, 1.62, 1.6300000000000001, 1.6400000000000001, 1.6500000000000001, 1.6600000000000001, 1.67, 1.68, 1.69, 1.7, 1.71, 1.72, 1.73, 1.74, 1.75, 1.76, 1.77, 1.78, 1.79, 1.8, 1.81, 1.82, 1.83, 1.84, 1.85, 1.86, 1.87, 1.8800000000000001, 1.8900000000000001, 1.9000000000000001, 1.9100000000000001, 1.92, 1.93, 1.94, 1.95, 1.96, 1.97, 1.98, 1.99, 2.0, 2.0100000000000002, 2.02, 2.0300000000000002, 2.04, 2.05, 2.06, 2.07, 2.08, 2.09, 2.1, 2.11, 2.12, 2.13, 2.14, 2.15, 2.16, 2.17, 2.18, 2.19, 2.2, 2.21, 2.22, 2.23, 2.24, 2.25, 2.2600000000000002, 2.27, 2.2800000000000002, 2.29, 2.3000000000000003, 2.31, 2.32, 2.33, 2.34, 2.35, 2.36, 2.37, 2.38, 2.39, 2.4, 2.41, 2.42, 2.43, 2.44, 2.45, 2.46, 2.47, 2.48, 2.49, 2.5, 2.5100000000000002, 2.52, 2.5300000000000002, 2.54, 2.5500000000000003, 2.56, 2.57, 2.58, 2.59, 2.6, 2.61, 2.62, 2.63, 2.64, 2.65, 2.66, 2.67, 2.68, 2.69, 2.7, 2.71, 2.72, 2.73, 2.74, 2.75, 2.7600000000000002, 2.77, 2.7800000000000002, 2.79, 2.8000000000000003, 2.81, 2.82, 2.83, 2.84, 2.85, 2.86, 2.87, 2.88, 2.89, 2.9, 2.91, 2.92, 2.93, 2.94, 2.95, 2.96, 2.97, 2.98, 2.99, 3.0], [0.0, 0.01, 0.02, 0.03, 0.04, 0.05, 0.060000000000000005, 0.07, 0.08, 0.09, 0.09999999999999999, 0.10999999999999999, 0.11999999999999998, 0.12999999999999998, 0.13999999999999999, 0.15, 0.16, 0.17, 0.18000000000000002, 0.19000000000000003, 0.20000000000000004, 0.21000000000000005, 0.22000000000000006, 0.23000000000000007, 0.24000000000000007, 0.25000000000000006, 0.26000000000000006, 0.2700000000000001, 0.2800000000000001, 0.2900000000000001, 0.3000000000000001, 0.3100000000000001, 0.3200000000000001, 0.3300000000000001, 0.34000000000000014, 0.35000000000000014, 0.36000000000000015, 0.37000000000000016, 0.38000000000000017, 0.3900000000000002, 0.4000000000000002, 0.4100000000000002, 0.4200000000000002, 0.4300000000000002, 0.4400000000000002, 0.45000000000000023, 0.46000000000000024, 0.47000000000000025, 0.48000000000000026, 0.49000000000000027, 0.5000000000000002, 0.5100000000000002, 0.5200000000000002, 0.5300000000000002, 0.5400000000000003, 0.5500000000000003, 0.5600000000000003, 0.5700000000000003, 0.5800000000000003, 0.5900000000000003, 0.6000000000000003, 0.6100000000000003, 0.6200000000000003, 0.6300000000000003, 0.6400000000000003, 0.6500000000000004, 0.6600000000000004, 0.6700000000000004, 0.6800000000000004, 0.6900000000000004, 0.7000000000000004, 0.7100000000000004, 0.7200000000000004, 0.7300000000000004, 0.7400000000000004, 0.7500000000000004, 0.7600000000000005, 0.7700000000000005, 0.7800000000000005, 0.7900000000000005, 0.8000000000000005, 0.8100000000000005, 0.8200000000000005, 0.8300000000000005, 0.8400000000000005, 0.8500000000000005, 0.8600000000000005, 0.8700000000000006, 0.8800000000000006, 0.8900000000000006, 0.9000000000000006, 0.9100000000000006, 0.9200000000000006, 0.9300000000000006, 0.9400000000000006, 0.9500000000000006, 0.9600000000000006, 0.9700000000000006, 0.9800000000000006, 0.9900000000000007, 1.0000000000000007, 1.0100000000000007, 1.0200000000000007, 1.0300000000000007, 1.0400000000000007, 1.0500000000000007, 1.0600000000000007, 1.0700000000000007, 1.0800000000000007, 1.0900000000000007, 1.1000000000000008, 1.1100000000000008, 1.1200000000000008, 1.1300000000000008, 1.1400000000000008, 1.1500000000000008, 1.1600000000000008, 1.1700000000000008, 1.1800000000000008, 1.1900000000000008, 1.2000000000000008, 1.2100000000000009, 1.2200000000000009, 1.2300000000000009, 1.2400000000000009, 1.2500000000000009, 1.260000000000001, 1.270000000000001, 1.280000000000001, 1.290000000000001, 1.300000000000001, 1.310000000000001, 1.320000000000001, 1.330000000000001, 1.340000000000001, 1.350000000000001, 1.360000000000001, 1.370000000000001, 1.380000000000001, 1.390000000000001, 1.400000000000001, 1.410000000000001, 1.420000000000001, 1.430000000000001, 1.440000000000001, 1.450000000000001, 1.460000000000001, 1.470000000000001, 1.480000000000001, 1.490000000000001, 1.500000000000001, 1.5100000000000011, 1.5200000000000011, 1.5300000000000011, 1.5400000000000011, 1.5500000000000012, 1.5600000000000012, 1.5700000000000012, 1.5800000000000012, 1.5900000000000012, 1.6000000000000012, 1.6100000000000012, 1.6200000000000012, 1.6300000000000012, 1.6400000000000012, 1.6500000000000012, 1.6600000000000013, 1.6700000000000013, 1.6800000000000013, 1.6900000000000013, 1.7000000000000013, 1.7100000000000013, 1.7200000000000013, 1.7300000000000013, 1.7400000000000013, 1.7500000000000013, 1.7600000000000013, 1.7700000000000014, 1.7800000000000014, 1.7900000000000014, 1.8000000000000014, 1.8100000000000014, 1.8200000000000014, 1.8300000000000014, 1.8400000000000014, 1.8500000000000014, 1.8600000000000014, 1.8700000000000014, 1.8800000000000014, 1.8900000000000015, 1.9000000000000015, 1.9100000000000015, 1.9200000000000015, 1.9300000000000015, 1.9400000000000015, 1.9500000000000015, 1.9600000000000015, 1.9700000000000015, 1.9800000000000015, 1.9900000000000015, 2.0000000000000013, 2.010000000000001, 2.020000000000001, 2.0300000000000007, 2.0400000000000005, 2.0500000000000003, 2.06, 2.07, 2.0799999999999996, 2.0899999999999994, 2.099999999999999, 2.109999999999999, 2.1199999999999988, 2.1299999999999986, 2.1399999999999983, 2.149999999999998, 2.159999999999998, 2.1699999999999977, 2.1799999999999975, 2.1899999999999973, 2.199999999999997, 2.209999999999997, 2.2199999999999966, 2.2299999999999964, 2.239999999999996, 2.249999999999996, 2.259999999999996, 2.2699999999999956, 2.2799999999999954, 2.289999999999995, 2.299999999999995, 2.3099999999999947, 2.3199999999999945, 2.3299999999999943, 2.339999999999994, 2.349999999999994, 2.3599999999999937, 2.3699999999999934, 2.3799999999999932, 2.389999999999993, 2.399999999999993, 2.4099999999999926, 2.4199999999999924, 2.429999999999992, 2.439999999999992, 2.4499999999999917, 2.4599999999999915, 2.4699999999999913, 2.479999999999991, 2.489999999999991, 2.4999999999999907, 2.5099999999999905, 2.5199999999999902, 2.52999999999999, 2.53999999999999, 2.5499999999999896, 2.5599999999999894, 2.569999999999989, 2.579999999999989, 2.5899999999999888, 2.5999999999999885, 2.6099999999999883, 2.619999999999988, 2.629999999999988, 2.6399999999999877, 2.6499999999999875, 2.6599999999999873, 2.669999999999987, 2.679999999999987, 2.6899999999999866, 2.6999999999999864, 2.709999999999986, 2.719999999999986, 2.7299999999999858, 2.7399999999999856, 2.7499999999999853, 2.759999999999985, 2.769999999999985, 2.7799999999999847, 2.7899999999999845, 2.7999999999999843, 2.809999999999984, 2.819999999999984, 2.8299999999999836, 2.8399999999999834, 2.849999999999983, 2.859999999999983, 2.869999999999983, 2.8799999999999826, 2.8899999999999824, 2.899999999999982, 2.909999999999982, 2.9199999999999817, 2.9299999999999815, 2.9399999999999813, 2.949999999999981, 2.959999999999981, 2.9699999999999807, 2.9799999999999804, 2.9899999999999802, 2.99999999999998]}]
  out "Step Response PID":cluster{"time":dbl[], dbl[]}[](graph)=[{"time"=[0.0, 0.01, 0.02, 0.03, 0.04, 0.05, 0.06, 0.07, 0.08, 0.09, 0.1, 0.11, 0.12, 0.13, 0.14, 0.15, 0.16, 0.17, 0.18, 0.19, 0.2, 0.21, 0.22, 0.23, 0.24, 0.25, 0.26, 0.27, 0.28, 0.29, 0.3, 0.31, 0.32, 0.33, 0.34, 0.35000000000000003, 0.36, 0.37, 0.38, 0.39, 0.4, 0.41000000000000003, 0.42, 0.43, 0.44, 0.45, 0.46, 0.47000000000000003, 0.48, 0.49, 0.5, 0.51, 0.52, 0.53, 0.54, 0.55, 0.56, 0.5700000000000001, 0.58, 0.59, 0.6, 0.61, 0.62, 0.63, 0.64, 0.65, 0.66, 0.67, 0.68, 0.6900000000000001, 0.7000000000000001, 0.71, 0.72, 0.73, 0.74, 0.75, 0.76, 0.77, 0.78, 0.79, 0.8, 0.81, 0.8200000000000001, 0.8300000000000001, 0.84, 0.85, 0.86, 0.87, 0.88, 0.89, 0.9, 0.91, 0.92, 0.93, 0.9400000000000001, 0.9500000000000001, 0.96, 0.97, 0.98, 0.99, 1.0, 1.01, 1.02, 1.03, 1.04, 1.05, 1.06, 1.07, 1.08, 1.09, 1.1, 1.11, 1.12, 1.1300000000000001, 1.1400000000000001, 1.1500000000000001, 1.16, 1.17, 1.18, 1.19, 1.2, 1.21, 1.22, 1.23, 1.24, 1.25, 1.26, 1.27, 1.28, 1.29, 1.3, 1.31, 1.32, 1.33, 1.34, 1.35, 1.36, 1.37, 1.3800000000000001, 1.3900000000000001, 1.4000000000000001, 1.41, 1.42, 1.43, 1.44, 1.45, 1.46, 1.47, 1.48, 1.49, 1.5, 1.51, 1.52, 1.53, 1.54, 1.55, 1.56, 1.57, 1.58, 1.59, 1.6, 1.61, 1.62, 1.6300000000000001, 1.6400000000000001, 1.6500000000000001, 1.6600000000000001, 1.67, 1.68, 1.69, 1.7, 1.71, 1.72, 1.73, 1.74, 1.75, 1.76, 1.77, 1.78, 1.79, 1.8, 1.81, 1.82, 1.83, 1.84, 1.85, 1.86, 1.87, 1.8800000000000001, 1.8900000000000001, 1.9000000000000001, 1.9100000000000001, 1.92, 1.93, 1.94, 1.95, 1.96, 1.97, 1.98, 1.99, 2.0, 2.0100000000000002, 2.02, 2.0300000000000002, 2.04, 2.05, 2.06, 2.07, 2.08, 2.09, 2.1, 2.11, 2.12, 2.13, 2.14, 2.15, 2.16, 2.17, 2.18, 2.19, 2.2, 2.21, 2.22, 2.23, 2.24, 2.25, 2.2600000000000002, 2.27, 2.2800000000000002, 2.29, 2.3000000000000003, 2.31, 2.32, 2.33, 2.34, 2.35, 2.36, 2.37, 2.38, 2.39, 2.4, 2.41, 2.42, 2.43, 2.44, 2.45, 2.46, 2.47, 2.48, 2.49, 2.5, 2.5100000000000002, 2.52, 2.5300000000000002, 2.54, 2.5500000000000003, 2.56, 2.57, 2.58, 2.59, 2.6, 2.61, 2.62, 2.63, 2.64, 2.65, 2.66, 2.67, 2.68, 2.69, 2.7, 2.71, 2.72, 2.73, 2.74, 2.75, 2.7600000000000002, 2.77, 2.7800000000000002, 2.79, 2.8000000000000003, 2.81, 2.82, 2.83, 2.84, 2.85, 2.86, 2.87, 2.88, 2.89, 2.9, 2.91, 2.92, 2.93, 2.94, 2.95, 2.96, 2.97, 2.98, 2.99, 3.0], [0.0, 0.0, 0.0, 0.0, 0.0, 0.0, 0.0, 0.0, 0.0, 0.0, 0.0, 0.0, 0.0, 0.0, 0.0, 0.0, 0.0, 0.0, 0.0, 0.0, 0.0, 0.0, 0.0, 0.0, 0.0, 0.0, 0.0, 0.0, 0.0, 0.0, 0.0, 0.0, 0.0, 0.0, 0.0, 0.0, 0.0, 0.0, 0.0, 0.0, 0.0, 0.0, 0.0, 0.0, 0.0, 0.0, 0.0, 0.0, 0.0, 0.0, 0.0, 0.0, 0.0, 0.0, 0.0, 0.0, 0.0, 0.0, 0.0, 0.0, 0.0, 0.0, 0.0, 0.0, 0.0, 0.0, 0.0, 0.0, 0.0, 0.0, 0.0, 0.0, 0.0, 0.0, 0.0, 0.0, 0.0, 0.0, 0.0, 0.0, 0.0, 0.0, 0.0, 0.0, 0.0, 0.0, 0.0, 0.0, 0.0, 0.0, 0.0, 0.0, 0.0, 0.0, 0.0, 0.0, 0.0, 0.0, 0.0, 0.0, 0.0, 0.0, 0.0, 0.0, 0.0, 0.0, 0.0, 0.0, 0.0, 0.0, 0.0, 0.0, 0.0, 0.0, 0.0, 0.0, 0.0, 0.0, 0.0, 0.0, 0.0, 0.0, 0.0, 0.0, 0.0, 0.0, 0.0, 0.0, 0.0, 0.0, 0.0, 0.0, 0.0, 0.0, 0.0, 0.0, 0.0, 0.0, 0.0, 0.0, 0.0, 0.0, 0.0, 0.0, 0.0, 0.0, 0.0, 0.0, 0.0, 0.0, 0.0, 0.0, 0.0, 0.0, 0.0, 0.0, 0.0, 0.0, 0.0, 0.0, 0.0, 0.0, 0.0, 0.0, 0.0, 0.0, 0.0, 0.0, 0.0, 0.0, 0.0, 0.0, 0.0, 0.0, 0.0, 0.0, 0.0, 0.0, 0.0, 0.0, 0.0, 0.0, 0.0, 0.0, 0.0, 0.0, 0.0, 0.0, 0.0, 0.0, 0.0, 0.0, 0.0, 0.0, 0.0, 0.0, 0.0, 0.0, 0.0, 0.0, 0.0, 0.0, 0.0, 0.0, 0.0, 0.0, 0.0, 0.0, 0.0, 0.0, 0.0, 0.0, 0.0, 0.0, 0.0, 0.0, 0.0, 0.0, 0.0, 0.0, 0.0, 0.0, 0.0, 0.0, 0.0, 0.0, 0.0, 0.0, 0.0, 0.0, 0.0, 0.0, 0.0, 0.0, 0.0, 0.0, 0.0, 0.0, 0.0, 0.0, 0.0, 0.0, 0.0, 0.0, 0.0, 0.0, 0.0, 0.0, 0.0, 0.0, 0.0, 0.0, 0.0, 0.0, 0.0, 0.0, 0.0, 0.0, 0.0, 0.0, 0.0, 0.0, 0.0, 0.0, 0.0, 0.0, 0.0, 0.0, 0.0, 0.0, 0.0, 0.0, 0.0, 0.0, 0.0, 0.0, 0.0, 0.0, 0.0, 0.0, 0.0, 0.0, 0.0, 0.0, 0.0, 0.0, 0.0, 0.0, 0.0, 0.0, 0.0, 0.0, 0.0, 0.0, 0.0, 0.0, 0.0, 0.0, 0.0, 0.0, 0.0]}, {"time"=[0.0, 0.01, 0.02, 0.03, 0.04, 0.05, 0.06, 0.07, 0.08, 0.09, 0.1, 0.11, 0.12, 0.13, 0.14, 0.15, 0.16, 0.17, 0.18, 0.19, 0.2, 0.21, 0.22, 0.23, 0.24, 0.25, 0.26, 0.27, 0.28, 0.29, 0.3, 0.31, 0.32, 0.33, 0.34, 0.35000000000000003, 0.36, 0.37, 0.38, 0.39, 0.4, 0.41000000000000003, 0.42, 0.43, 0.44, 0.45, 0.46, 0.47000000000000003, 0.48, 0.49, 0.5, 0.51, 0.52, 0.53, 0.54, 0.55, 0.56, 0.5700000000000001, 0.58, 0.59, 0.6, 0.61, 0.62, 0.63, 0.64, 0.65, 0.66, 0.67, 0.68, 0.6900000000000001, 0.7000000000000001, 0.71, 0.72, 0.73, 0.74, 0.75, 0.76, 0.77, 0.78, 0.79, 0.8, 0.81, 0.8200000000000001, 0.8300000000000001, 0.84, 0.85, 0.86, 0.87, 0.88, 0.89, 0.9, 0.91, 0.92, 0.93, 0.9400000000000001, 0.9500000000000001, 0.96, 0.97, 0.98, 0.99, 1.0, 1.01, 1.02, 1.03, 1.04, 1.05, 1.06, 1.07, 1.08, 1.09, 1.1, 1.11, 1.12, 1.1300000000000001, 1.1400000000000001, 1.1500000000000001, 1.16, 1.17, 1.18, 1.19, 1.2, 1.21, 1.22, 1.23, 1.24, 1.25, 1.26, 1.27, 1.28, 1.29, 1.3, 1.31, 1.32, 1.33, 1.34, 1.35, 1.36, 1.37, 1.3800000000000001, 1.3900000000000001, 1.4000000000000001, 1.41, 1.42, 1.43, 1.44, 1.45, 1.46, 1.47, 1.48, 1.49, 1.5, 1.51, 1.52, 1.53, 1.54, 1.55, 1.56, 1.57, 1.58, 1.59, 1.6, 1.61, 1.62, 1.6300000000000001, 1.6400000000000001, 1.6500000000000001, 1.6600000000000001, 1.67, 1.68, 1.69, 1.7, 1.71, 1.72, 1.73, 1.74, 1.75, 1.76, 1.77, 1.78, 1.79, 1.8, 1.81, 1.82, 1.83, 1.84, 1.85, 1.86, 1.87, 1.8800000000000001, 1.8900000000000001, 1.9000000000000001, 1.9100000000000001, 1.92, 1.93, 1.94, 1.95, 1.96, 1.97, 1.98, 1.99, 2.0, 2.0100000000000002, 2.02, 2.0300000000000002, 2.04, 2.05, 2.06, 2.07, 2.08, 2.09, 2.1, 2.11, 2.12, 2.13, 2.14, 2.15, 2.16, 2.17, 2.18, 2.19, 2.2, 2.21, 2.22, 2.23, 2.24, 2.25, 2.2600000000000002, 2.27, 2.2800000000000002, 2.29, 2.3000000000000003, 2.31, 2.32, 2.33, 2.34, 2.35, 2.36, 2.37, 2.38, 2.39, 2.4, 2.41, 2.42, 2.43, 2.44, 2.45, 2.46, 2.47, 2.48, 2.49, 2.5, 2.5100000000000002, 2.52, 2.5300000000000002, 2.54, 2.5500000000000003, 2.56, 2.57, 2.58, 2.59, 2.6, 2.61, 2.62, 2.63, 2.64, 2.65, 2.66, 2.67, 2.68, 2.69, 2.7, 2.71, 2.72, 2.73, 2.74, 2.75, 2.7600000000000002, 2.77, 2.7800000000000002, 2.79, 2.8000000000000003, 2.81, 2.82, 2.83, 2.84, 2.85, 2.86, 2.87, 2.88, 2.89, 2.9, 2.91, 2.92, 2.93, 2.94, 2.95, 2.96, 2.97, 2.98, 2.99, 3.0], [1.0, 1.0, 1.0, 1.0, 1.0, 1.0, 1.0, 1.0, 1.0, 1.0, 1.0, 1.0, 1.0, 1.0, 1.0, 1.0, 1.0, 1.0, 1.0, 1.0, 1.0, 1.0, 1.0, 1.0, 1.0, 1.0, 1.0, 1.0, 1.0, 1.0, 1.0, 1.0, 1.0, 1.0, 1.0, 1.0, 1.0, 1.0, 1.0, 1.0, 1.0, 1.0, 1.0, 1.0, 1.0, 1.0, 1.0, 1.0, 1.0, 1.0, 1.0, 1.0, 1.0, 1.0, 1.0, 1.0, 1.0, 1.0, 1.0, 1.0, 1.0, 1.0, 1.0, 1.0, 1.0, 1.0, 1.0, 1.0, 1.0, 1.0, 1.0, 1.0, 1.0, 1.0, 1.0, 1.0, 1.0, 1.0, 1.0, 1.0, 1.0, 1.0, 1.0, 1.0, 1.0, 1.0, 1.0, 1.0, 1.0, 1.0, 1.0, 1.0, 1.0, 1.0, 1.0, 1.0, 1.0, 1.0, 1.0, 1.0, 1.0, 1.0, 1.0, 1.0, 1.0, 1.0, 1.0, 1.0, 1.0, 1.0, 1.0, 1.0, 1.0, 1.0, 1.0, 1.0, 1.0, 1.0, 1.0, 1.0, 1.0, 1.0, 1.0, 1.0, 1.0, 1.0, 1.0, 1.0, 1.0, 1.0, 1.0, 1.0, 1.0, 1.0, 1.0, 1.0, 1.0, 1.0, 1.0, 1.0, 1.0, 1.0, 1.0, 1.0, 1.0, 1.0, 1.0, 1.0, 1.0, 1.0, 1.0, 1.0, 1.0, 1.0, 1.0, 1.0, 1.0, 1.0, 1.0, 1.0, 1.0, 1.0, 1.0, 1.0, 1.0, 1.0, 1.0, 1.0, 1.0, 1.0, 1.0, 1.0, 1.0, 1.0, 1.0, 1.0, 1.0, 1.0, 1.0, 1.0, 1.0, 1.0, 1.0, 1.0, 1.0, 1.0, 1.0, 1.0, 1.0, 1.0, 1.0, 1.0, 1.0, 1.0, 1.0, 1.0, 1.0, 1.0, 1.0, 1.0, 1.0, 1.0, 1.0, 1.0, 1.0, 1.0, 1.0, 1.0, 1.0, 1.0, 1.0, 1.0, 1.0, 1.0, 1.0, 1.0, 1.0, 1.0, 1.0, 1.0, 1.0, 1.0, 1.0, 1.0, 1.0, 1.0, 1.0, 1.0, 1.0, 1.0, 1.0, 1.0, 1.0, 1.0, 1.0, 1.0, 1.0, 1.0, 1.0, 1.0, 1.0, 1.0, 1.0, 1.0, 1.0, 1.0, 1.0, 1.0, 1.0, 1.0, 1.0, 1.0, 1.0, 1.0, 1.0, 1.0, 1.0, 1.0, 1.0, 1.0, 1.0, 1.0, 1.0, 1.0, 1.0, 1.0, 1.0, 1.0, 1.0, 1.0, 1.0, 1.0, 1.0, 1.0, 1.0, 1.0, 1.0, 1.0, 1.0, 1.0, 1.0, 1.0, 1.0, 1.0, 1.0, 1.0, 1.0, 1.0, 1.0, 1.0, 1.0, 1.0, 1.0, 1.0, 1.0, 1.0, 1.0, 1.0, 1.0, 1.0, 1.0]}]
  out "Root Locus PID":cluster{dbl[], dbl[]}[](graph)
  in  "G":T1 {"transfer function(s)"."delay" format="%.4f"; "transfer function(s)"."Denominator" format="%#_3g"; "transfer function(s)"."Numerator" format="%#_3g"; "properties"."Sampling Time" format="%#.6p"; "properties"."Output Delays" format="%.4f"; "properties"."Input Delays" format="%.4f"}
  out "Derivative time [s] (Td)":dbl
  out "Integral time [s] (Ti)":dbl=inf
  out "Proportional Gain (Kc)":dbl
  in  "choose":string(combo)="PID"
  out "PID":dbl[](array[numeric])=[3.1578947368421058, 2.3749999999999996, 0.5937499999999999]
  out "L":dbl=1.1874999999999998
  out "T":dbl=3.0625000000000004
  out "k":dbl=0.98
  in  "t":dbl[](array[numeric])=[0.0, 0.5, 1.0, 1.5, 2.0, 2.5, 3.0, 3.5, 4.0, 4.5, 5.0, 5.5, 6.0, 7.0]
  in  "y":dbl[](array[numeric])=[0.0, 0.02, 0.05, 0.16, 0.28, 0.42, 0.58, 0.7, 0.8, 0.86, 0.92, 0.95, 0.97, 0.98]
  in  "u":dbl[](array[numeric])=[1.0]
  # "KP"
  # "TI"
  # "TD"
  # "############################################################################################################################################################################################"
  # "ZIEGELER 2ND METHOD"
  # "THE ANS FOR TABLE"
  # "#\n#\n#\n#\n#\n#\n#\n#\n#\n#\n#\n#\n#\n#"
  # "design"
  # "PD"
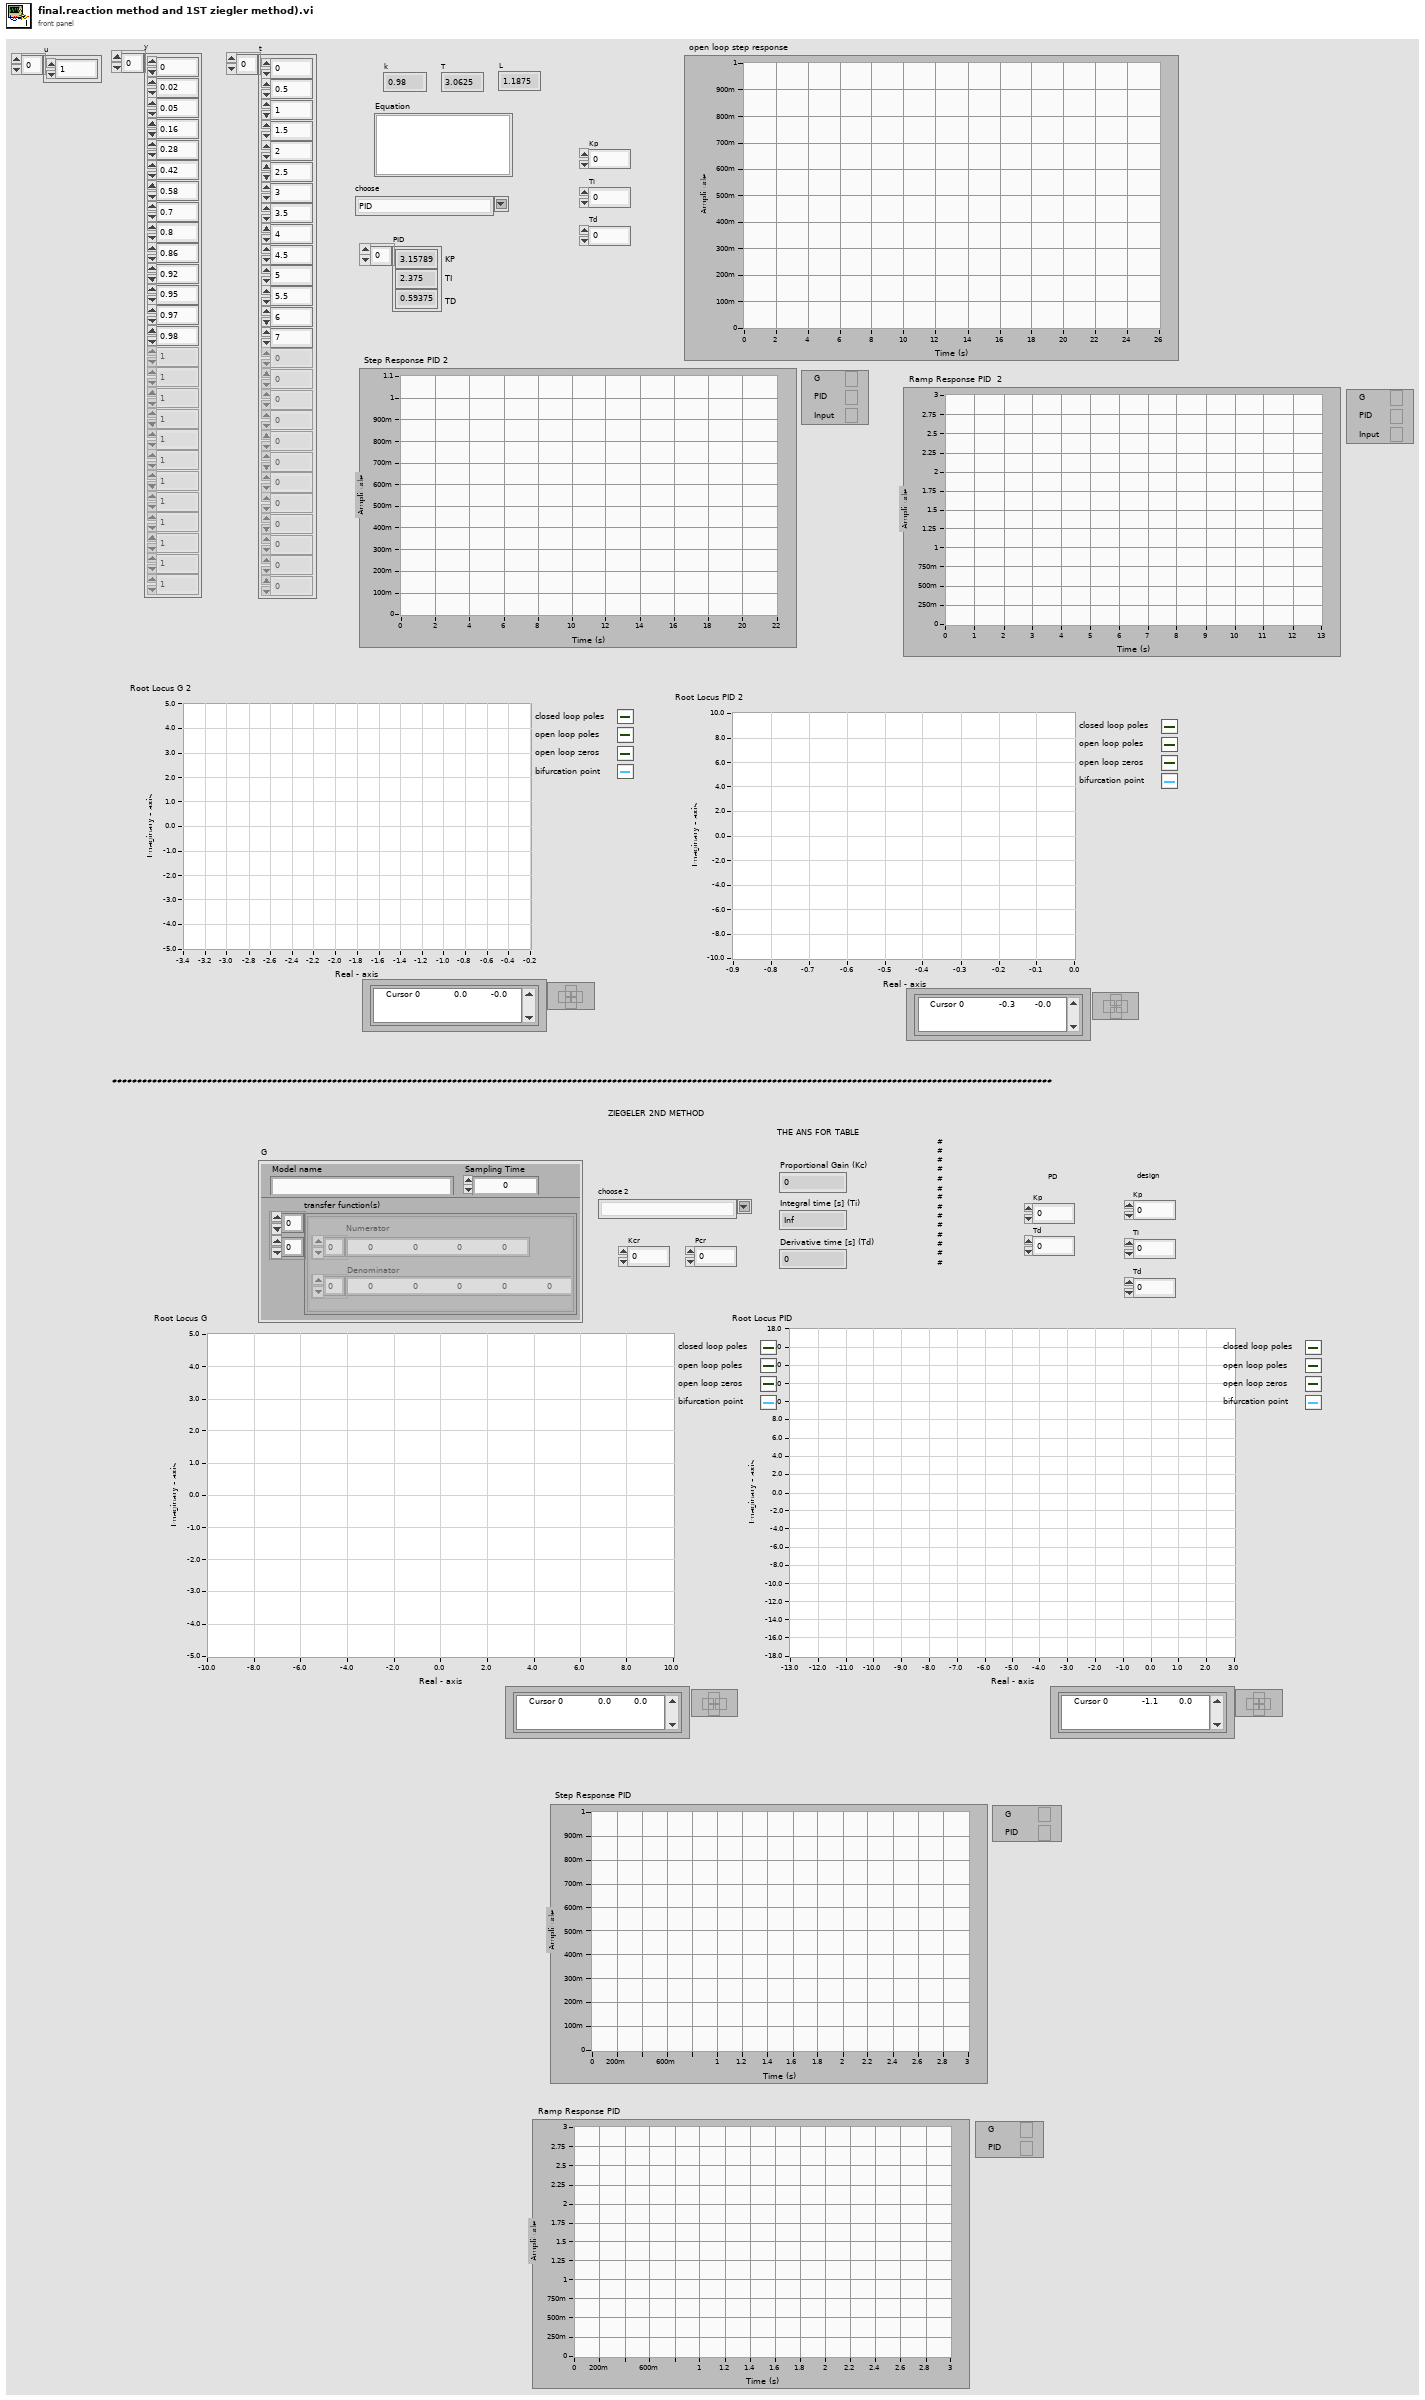
[diagram p1: front panel]
types:
  T1 = typedef "NI_LinSys_Model Typedefs.lvlib/CD Transfer Function Model (MIMO).ctl" = cluster{"properties":T2, "transfer function(s)":T3[][]}
  T2 = typedef "NI_LinSys_Model Typedefs.lvlib/CD General Elements.ctl" = cluster{"Model name":string, "Input names":string[], "Output names":string[], "Input Delays":dbl[], "Output Delays":dbl[], "Sampling Time":dbl, "Notes":string}
  T3 = typedef "NI_LinSys_Model Typedefs.lvlib/CD Transfer Function Model (SISO).ctl" = cluster{"Numerator":dbl[], "Denominator":dbl[], "delay":dbl}
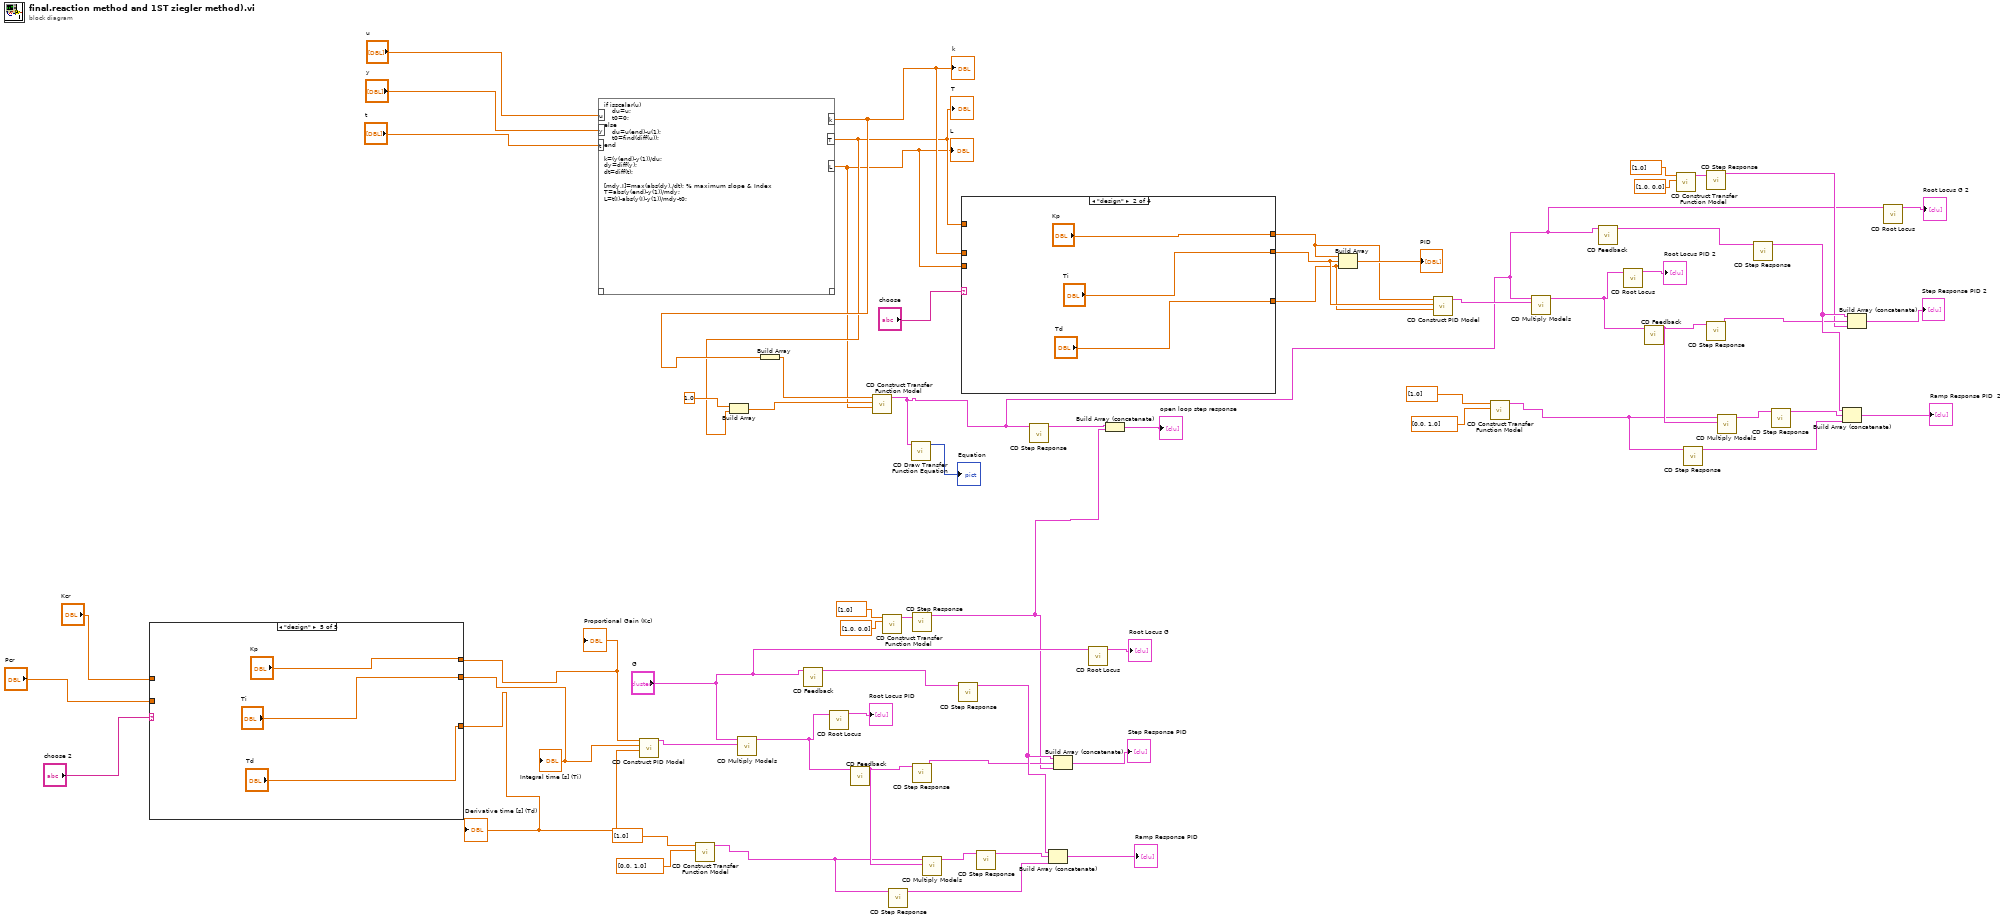
[diagram p0: block diagram]
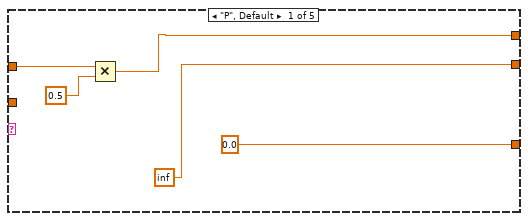
[diagram p2: hidden frame]
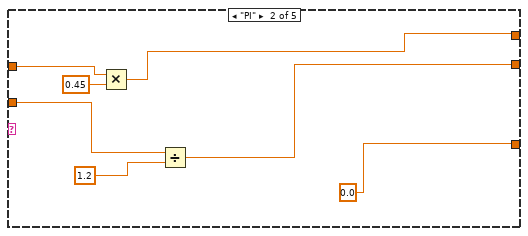
[diagram p3: hidden frame]
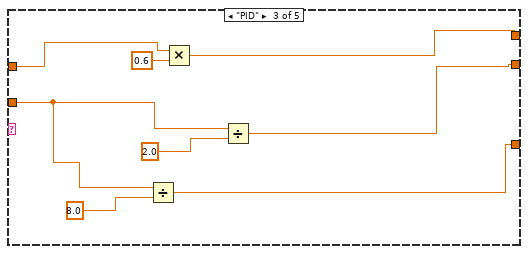
[diagram p4: hidden frame]
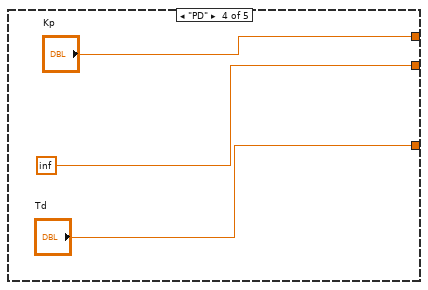
[diagram p5: hidden frame]
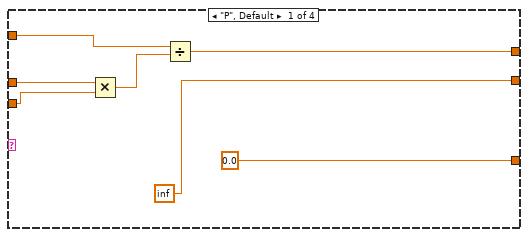
[diagram p6: hidden frame]
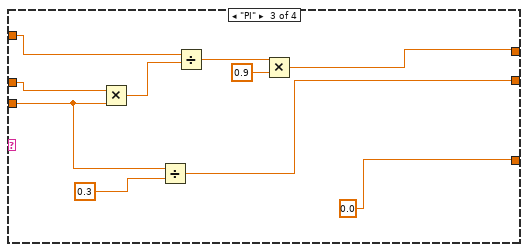
[diagram p7: hidden frame]
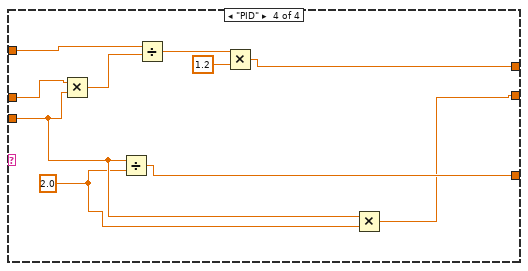
[diagram p8: hidden frame]
diagram:
  n1 = case shown="\"design\"" "choose 2" {
    tunnel: [w67 w72 w79 "Kp" "Kp"] -> w42
    tunnel: [inf w75 w80 inf "Ti"] -> w41
    tunnel: [0.0 ("element") 0.0 ("element") w78 "Td" "Td"] -> w40
    tunnel: "Kcr" -> [w68 w73 w83 _ _]
    tunnel: "Pcr" -> [_ w71 w81 _ _]
    frame "P", Default {
      n2 = Multiply(x=w68, y=0.5) -> (x*y=w67:dbl)
    }
    frame "PI" {
      n3 = Multiply(x=w73, y=0.45) -> (x*y=w72:dbl)
      n4 = Divide(x=w71, y=1.2) -> (x/y=w75:dbl)
    }
    frame "PID" {
      n5 = Divide(x=w81, y=8.0) -> (x/y=w78:dbl)
      n6 = Multiply(x=w83, y=0.6) -> (x*y=w79:dbl)
      n7 = Divide(x=w81, y=2.0) -> (x/y=w80:dbl)
    }
    frame "PD" {
    }
    frame "design" {
    }
  }
  "Proportional Gain (Kc)" <- w42
  "Integral time [s] (Ti)" <- w41
  "Derivative time [s] (Td)" <- w40
  n8 = script code="if isscalar(u)\n    du=u;\n    t0=0;\nelse\n    du=u(end)-u(1);\n    t0=find(diff(u));\nend\n\nk=(y(end)-y(1))/du;\ndy=diff(y);\ndt=diff(t);\n\n[mdy,I]=max(abs(dy)./dt); % maximum slope & Index\nT=abs(y(end)-y(1))/mdy;\nL=t(I)-abs(y(I)-y(1))/mdy-t0;"("u"="u", "y"="y", "t"="t") -> ("k"=w27:dbl, "T"=w26:dbl, "L"=w25:dbl)  [unwired: 1 in, 1 out]
  "k" <- w27
  "T" <- w26
  "L" <- w25
  n9 = call-poly <vilib>:"CD Construct PID Model.vi"("Derivative time [s] (Td)"=w40, "Integral time [s] (Ti)"=w41, "Proportional Gain (Kc)"=w42) -> ("Transfer Function Model"=w62:T1)  [unwired: 7 in, 1 out]
  n10 = call-poly <vilib>:"CD Construct Transfer Function Model.vi"("Denominator"=dbl[] [0.0, 1.0], "Numerator"=dbl[] [1.0]) -> ("Transfer Function Model"=w47:T1)  [unwired: 8 in, 1 out]
  n11 = Build Array(1.0 ("element"), w26) -> (w35:dbl[])
  n12 = call-poly <vilib>:"CD Multiply Models.vi"("Model 2"=w62, "Model 1"="G") -> ("Model Out"=w60:T1)  [unwired: 8 in, 1 out]
  n13 = Build Array(w27) -> (w33:dbl[])
  n14 = call-poly <vilib>:"CD Feedback.vi"("Model 1"="G") -> ("Closed-Loop Model"=w44:T1)  [unwired: 9 in, 1 out]
  n15 = call-poly <vilib>:"CD Root Locus.vi"("Transfer Function Model"=w60) -> ("Root Locus Graph"=→"Root Locus PID":cluster{dbl[], dbl[]}[])  [unwired: 7 in, 3 out]
  n16 = call-poly <vilib>:"CD Feedback.vi"("Model 1"=w60) -> ("Closed-Loop Model"=w57:T1)  [unwired: 9 in, 1 out]
  n17 = call-poly <vilib>:"CD Construct Transfer Function Model.vi"("Delay"=w25, "Denominator"=w35, "Numerator"=w33) -> ("Transfer Function Model"=w4:T1)  [unwired: 7 in, 1 out]
  n18 = call-poly <vilib>:"CD Construct Transfer Function Model.vi"("Denominator"=dbl[] [1.0, 0.0], "Numerator"=dbl[] [1.0]) -> ("Transfer Function Model"=w48:T1)  [unwired: 8 in, 1 out]
  n19 = call-poly <vilib>:"CD Step Response.vi"("Transfer Function Model"=w47) -> ("Step Response Graph"=w46:cluster{"time":dbl[], dbl[]}[])  [unwired: 8 in, 2 out]
  n20 = call-poly <vilib>:"CD Draw Transfer Function Equation.vi"("Transfer Function Model"=w4) -> ("Equation"=→"Equation":picture)  [unwired: 8 in, 2 out]
  n21 = call-poly <vilib>:"CD Step Response.vi"("Transfer Function Model"=w48) -> ("Step Response Graph"=w30:cluster{"time":dbl[], dbl[]}[])  [unwired: 8 in, 2 out]
  n22 = call-poly <vilib>:"CD Step Response.vi"("Transfer Function Model"=w57) -> ("Step Response Graph"=w51:cluster{"time":dbl[], dbl[]}[])  [unwired: 8 in, 2 out]
  n23 = call-poly <vilib>:"CD Multiply Models.vi"("Model 2"=w57, "Model 1"=w47) -> ("Model Out"=w56:T1)  [unwired: 8 in, 1 out]
  n24 = call-poly <vilib>:"CD Step Response.vi"("Transfer Function Model"=w44) -> ("Step Response Graph"=w52:cluster{"time":dbl[], dbl[]}[])  [unwired: 8 in, 2 out]
  n25 = case shown="\"design\"" "choose" {
    tunnel: w27 -> [w98 _ w109 w117]
    tunnel: w25 -> [w97 _ w104 w116]
    tunnel: w26 -> [w96 _ w110 w118]
    tunnel: [w94 "Kp" w106 w112] -> w3
    tunnel: [inf "Ti" w102 w113] -> w2
    tunnel: [0.0 ("element") "Td" 0.0 ("element") w114] -> w1
    frame "P", Default {
      n26 = Multiply(x=w98, y=w97) -> (x*y=w95:dbl)
      n27 = Divide(x=w96, y=w95) -> (x/y=w94:dbl)
    }
    frame "design" {
    }
    frame "PI" {
      n28 = Multiply(x=w109, y=w104) -> (x*y=w111:dbl)
      n29 = Divide(x=w104, y=0.3) -> (x/y=w102:dbl)
      n30 = Divide(x=w110, y=w111) -> (x/y=w108:dbl)
      n31 = Multiply(x=w108, y=0.9) -> (x*y=w106:dbl)
    }
    frame "PID" {
      w115 = 2.0 ("y")
      n32 = Multiply(x=w117, y=w116) -> (x*y=w121:dbl)
      n33 = Divide(x=w116, y=w115) -> (x/y=w114:dbl)
      n34 = Divide(x=w118, y=w121) -> (x/y=w120:dbl)
      n35 = Multiply(x=w120, y=1.2) -> (x*y=w112:dbl)
      n36 = Multiply(x=w116, y=w115) -> (x*y=w113:dbl)
    }
  }
  n37 = call-poly <vilib>:"CD Step Response.vi"("Transfer Function Model"=w56) -> ("Step Response Graph"=w54:cluster{"time":dbl[], dbl[]}[])  [unwired: 8 in, 2 out]
  n38 = call-poly <vilib>:"CD Step Response.vi"("Transfer Function Model"=w4) -> ("Step Response Graph"=w32:cluster{"time":dbl[], dbl[]}[])  [unwired: 8 in, 2 out]
  n39 = Build Array (concatenate)(w52, w54, w46) -> (→"Ramp Response PID":cluster{"time":dbl[], dbl[]}[])
  n40 = Build Array (concatenate)(w52, w51, w30) -> (→"Step Response PID":cluster{"time":dbl[], dbl[]}[])
  n41 = call-poly <vilib>:"CD Root Locus.vi"("Transfer Function Model"="G") -> ("Root Locus Graph"=→"Root Locus G":cluster{dbl[], dbl[]}[])  [unwired: 7 in, 3 out]
  n42 = Build Array (concatenate)(w32, w30) -> (→"open loop step response":cluster{"time":dbl[], dbl[]}[])
  n43 = Build Array(w3, w2, w1) -> (→"PID":dbl[])
  n44 = call-poly <vilib>:"CD Construct PID Model.vi"("Derivative time [s] (Td)"=w1, "Integral time [s] (Ti)"=w2, "Proportional Gain (Kc)"=w3) -> ("Transfer Function Model"=w5:T1)  [unwired: 7 in, 1 out]
  n45 = call-poly <vilib>:"CD Construct Transfer Function Model.vi"("Denominator"=dbl[] [0.0, 1.0], "Numerator"=dbl[] [1.0]) -> ("Transfer Function Model"=w10:T1)  [unwired: 8 in, 1 out]
  n46 = call-poly <vilib>:"CD Multiply Models.vi"("Model 2"=w5, "Model 1"=w4) -> ("Model Out"=w23:T1)  [unwired: 8 in, 1 out]
  n47 = call-poly <vilib>:"CD Feedback.vi"("Model 1"=w4) -> ("Closed-Loop Model"=w7:T1)  [unwired: 9 in, 1 out]
  n48 = call-poly <vilib>:"CD Root Locus.vi"("Transfer Function Model"=w23) -> ("Root Locus Graph"=→"Root Locus PID 2":cluster{dbl[], dbl[]}[])  [unwired: 7 in, 3 out]
  n49 = call-poly <vilib>:"CD Feedback.vi"("Model 1"=w23) -> ("Closed-Loop Model"=w20:T1)  [unwired: 9 in, 1 out]
  n50 = call-poly <vilib>:"CD Construct Transfer Function Model.vi"("Denominator"=dbl[] [1.0, 0.0], "Numerator"=dbl[] [1.0]) -> ("Transfer Function Model"=w11:T1)  [unwired: 8 in, 1 out]
  n51 = call-poly <vilib>:"CD Step Response.vi"("Transfer Function Model"=w10) -> ("Step Response Graph"=w9:cluster{"time":dbl[], dbl[]}[])  [unwired: 8 in, 2 out]
  n52 = call-poly <vilib>:"CD Step Response.vi"("Transfer Function Model"=w11) -> ("Step Response Graph"=w6:cluster{"time":dbl[], dbl[]}[])  [unwired: 8 in, 2 out]
  n53 = call-poly <vilib>:"CD Step Response.vi"("Transfer Function Model"=w20) -> ("Step Response Graph"=w14:cluster{"time":dbl[], dbl[]}[])  [unwired: 8 in, 2 out]
  n54 = call-poly <vilib>:"CD Multiply Models.vi"("Model 2"=w20, "Model 1"=w10) -> ("Model Out"=w19:T1)  [unwired: 8 in, 1 out]
  n55 = call-poly <vilib>:"CD Step Response.vi"("Transfer Function Model"=w7) -> ("Step Response Graph"=w15:cluster{"time":dbl[], dbl[]}[])  [unwired: 8 in, 2 out]
  n56 = call-poly <vilib>:"CD Step Response.vi"("Transfer Function Model"=w19) -> ("Step Response Graph"=w17:cluster{"time":dbl[], dbl[]}[])  [unwired: 8 in, 2 out]
  n57 = Build Array (concatenate)(w15, w17, w9) -> (→"Ramp Response PID  2":cluster{"time":dbl[], dbl[]}[])
  n58 = Build Array (concatenate)(w15, w14, w6) -> (→"Step Response PID 2":cluster{"time":dbl[], dbl[]}[])
  n59 = call-poly <vilib>:"CD Root Locus.vi"("Transfer Function Model"=w4) -> ("Root Locus Graph"=→"Root Locus G 2":cluster{dbl[], dbl[]}[])  [unwired: 7 in, 3 out]
